vi "진짜 최종.vi"() -> ()   [LabVIEW 2016]
uses:
  <vilib>/DAQmx/write.llb/DAQmx Write (Digital 1D U32 1Chan NSamp).vi
  <vilib>/DAQmx/read.llb/DAQmx Read (Analog 1D Wfm NChan NSamp).vi
  <vilib>/DAQmx/create/channels.llb/DAQmx Create Channel (DO-Digital Output).vi
  <vilib>/DAQmx/configure/timing.llb/DAQmx Timing (Sample Clock).vi
  <vilib>/DAQmx/create/channels.llb/DAQmx Create Channel (AI-Acceleration-Accelerometer).vi
  <vilib>/DAQmx/miscellaneous.llb/DAQmx Fill In Error Info.vi
panel:
  out "Elapsed Time (s) 9":dbl caption="대기상태 경과시간"
  out "1세트점수":i32
  out "0세트점수":i32
  out "몇번째 경기":i32
  out "1터치횟수":i32
  out "0터치횟수":i32
  out "player 1":bool
  out "player 2":bool
  out "0현점수":i32
  out "1현점수":i32
  out "0번 터치":bool
  out "1번 터치":bool
  out "Elapsed Time (s) 8":dbl caption="0 터치인식대기"
  out "Elapsed Time (s) 7":dbl caption="1 터치인식대기"
  out "Elapsed Time (s) 6":dbl caption="1리시브"
  out "Elapsed Time (s)":dbl caption="0리시브"
  out "Elapsed Time (s) 5":dbl caption="0세트승리"
  out "Elapsed Time (s) 4":dbl caption="0번 승리 경과"
  out "Elapsed Time (s) 3":dbl caption="1세트승리"
  out "Elapsed Time (s) 2":dbl caption="1번 승리 경과"
  in  "RESET":bool
  # "HA"
  # "JIWON"
  # "2초 reset"
  # "2초 reset"
  # "2초 reset"
  # "0.05초 reset"
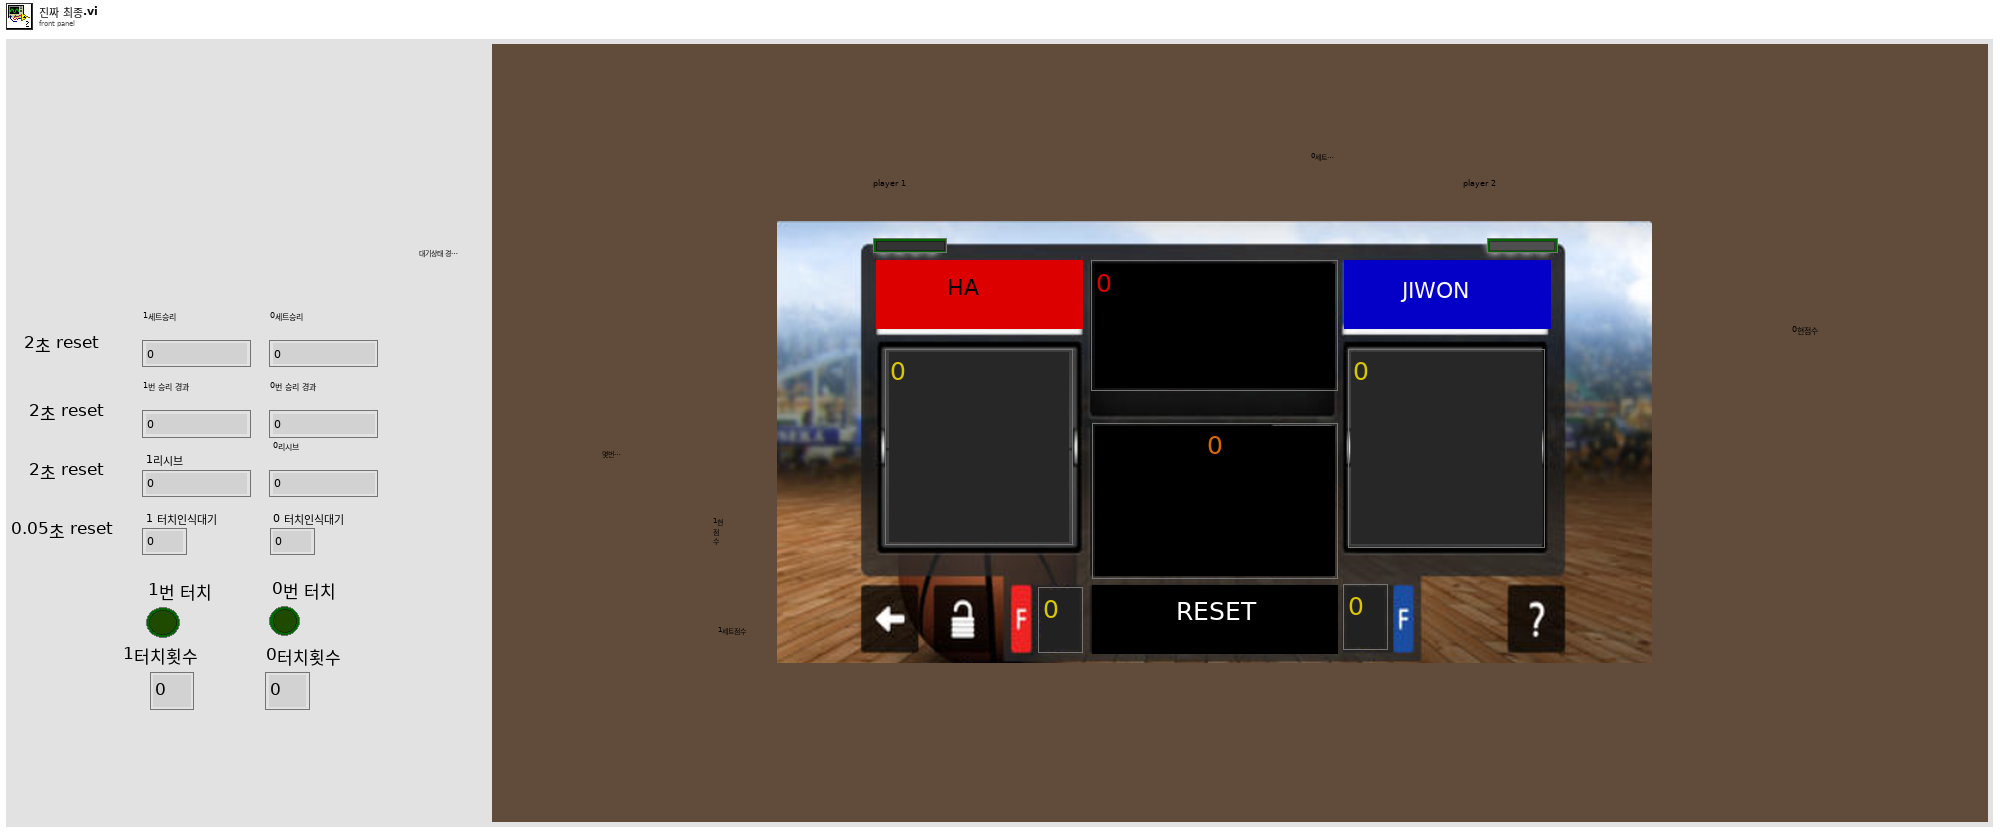
[diagram p1: front panel]
types:
  T1 = typedef "컨트롤 2.ctl" = enum16{"경기끝!", "1세트승리", "0세트승리", "0리시브", "1리시브", "대기", "1번터치", "0번터치", "서브교체", "1번승리", "0번승리"}
  T2 = cluster{"점수":i32[], "몇번째 경기":i32, "LED0":bool, "LED1":bool, "1번터치 횟수":i32, "0현점수":i32, "1현점수":i32, "0번터치 횟수":i32, "0세트점수":i32, "1세트점수":i32, "경과시간":i32, "0세트 이진수점수":u32[], "1세트 이진수점수 ":u32[], "LED1차례":u32[], "LED0차례":u32[]}
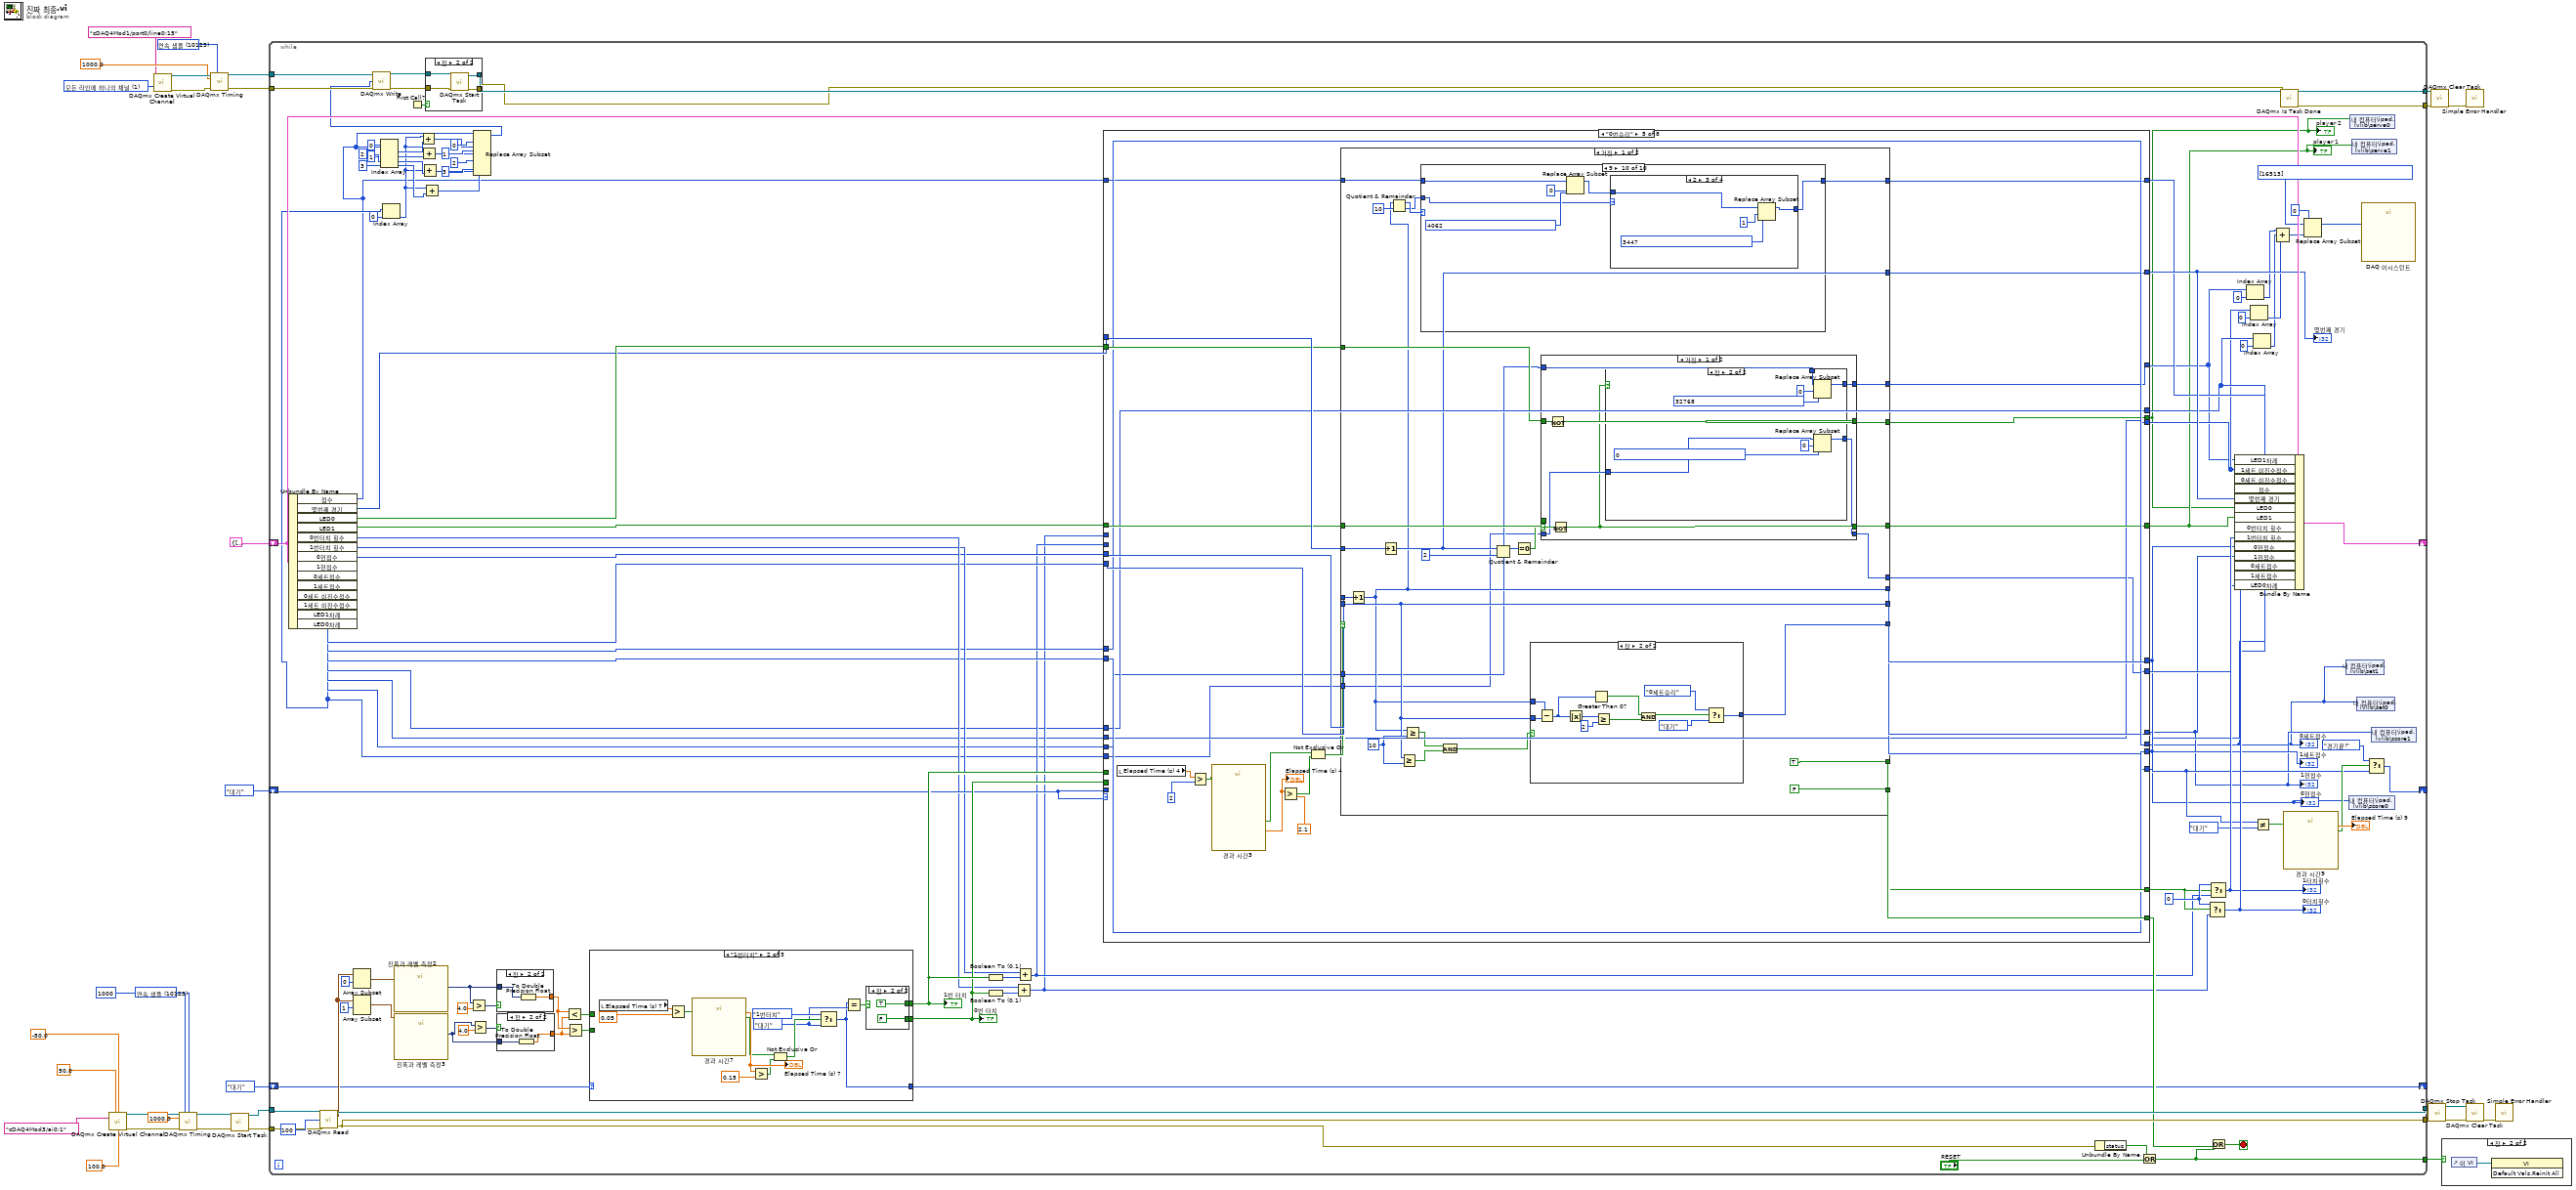
[diagram p0: block diagram]
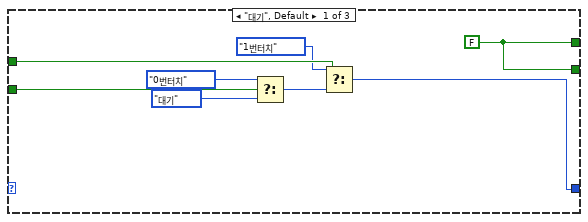
[diagram p2: hidden frame]
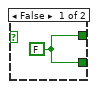
[diagram p3: hidden frame]
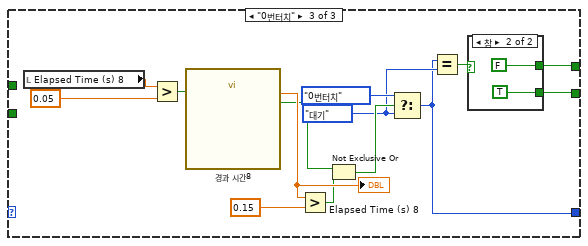
[diagram p4: hidden frame]
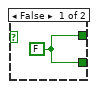
[diagram p5: hidden frame]
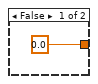
[diagram p6: hidden frame]
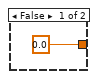
[diagram p7: hidden frame]
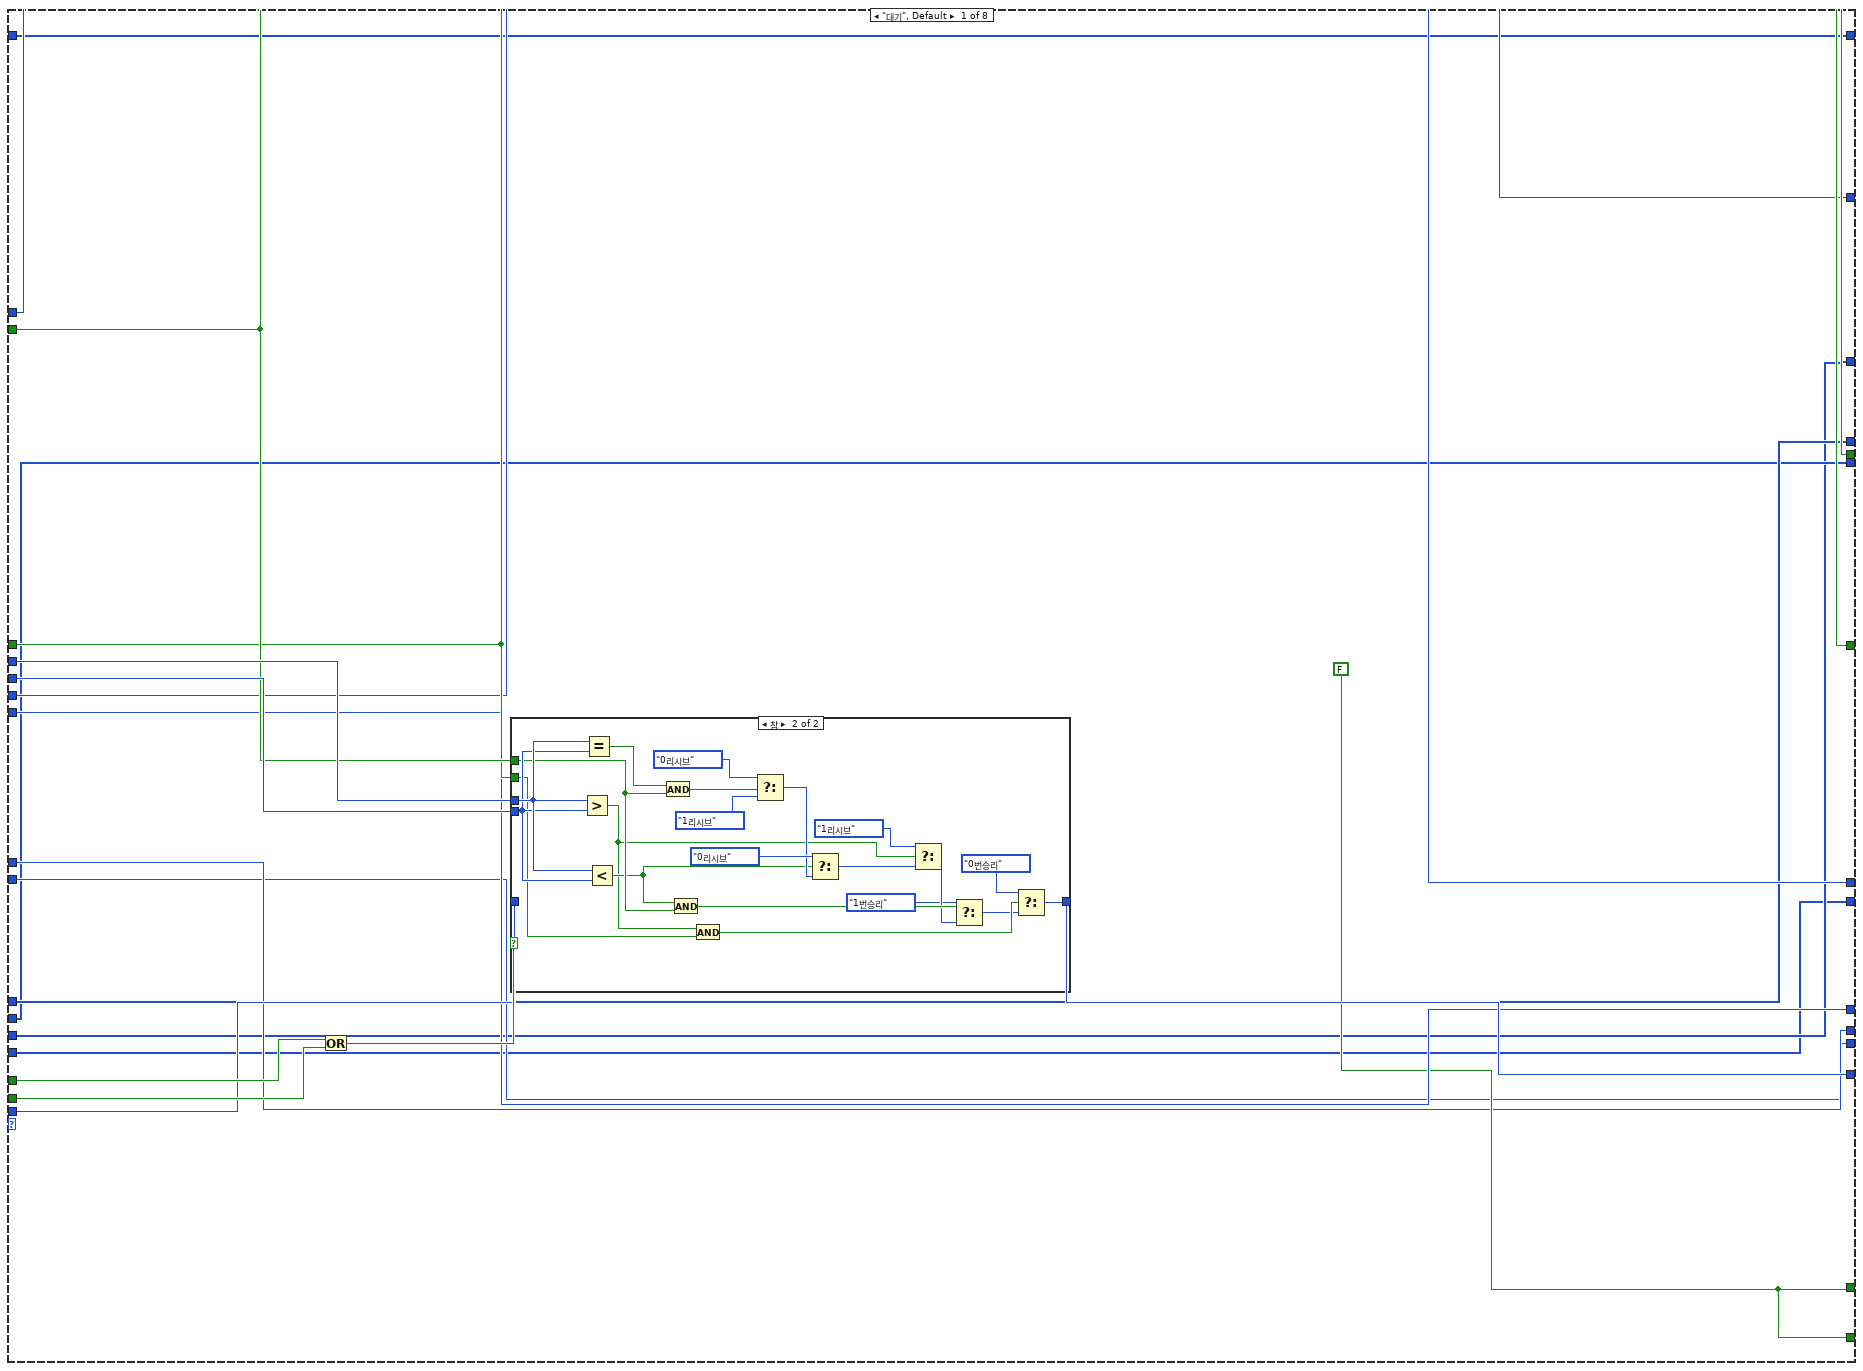
[diagram p8: hidden frame]
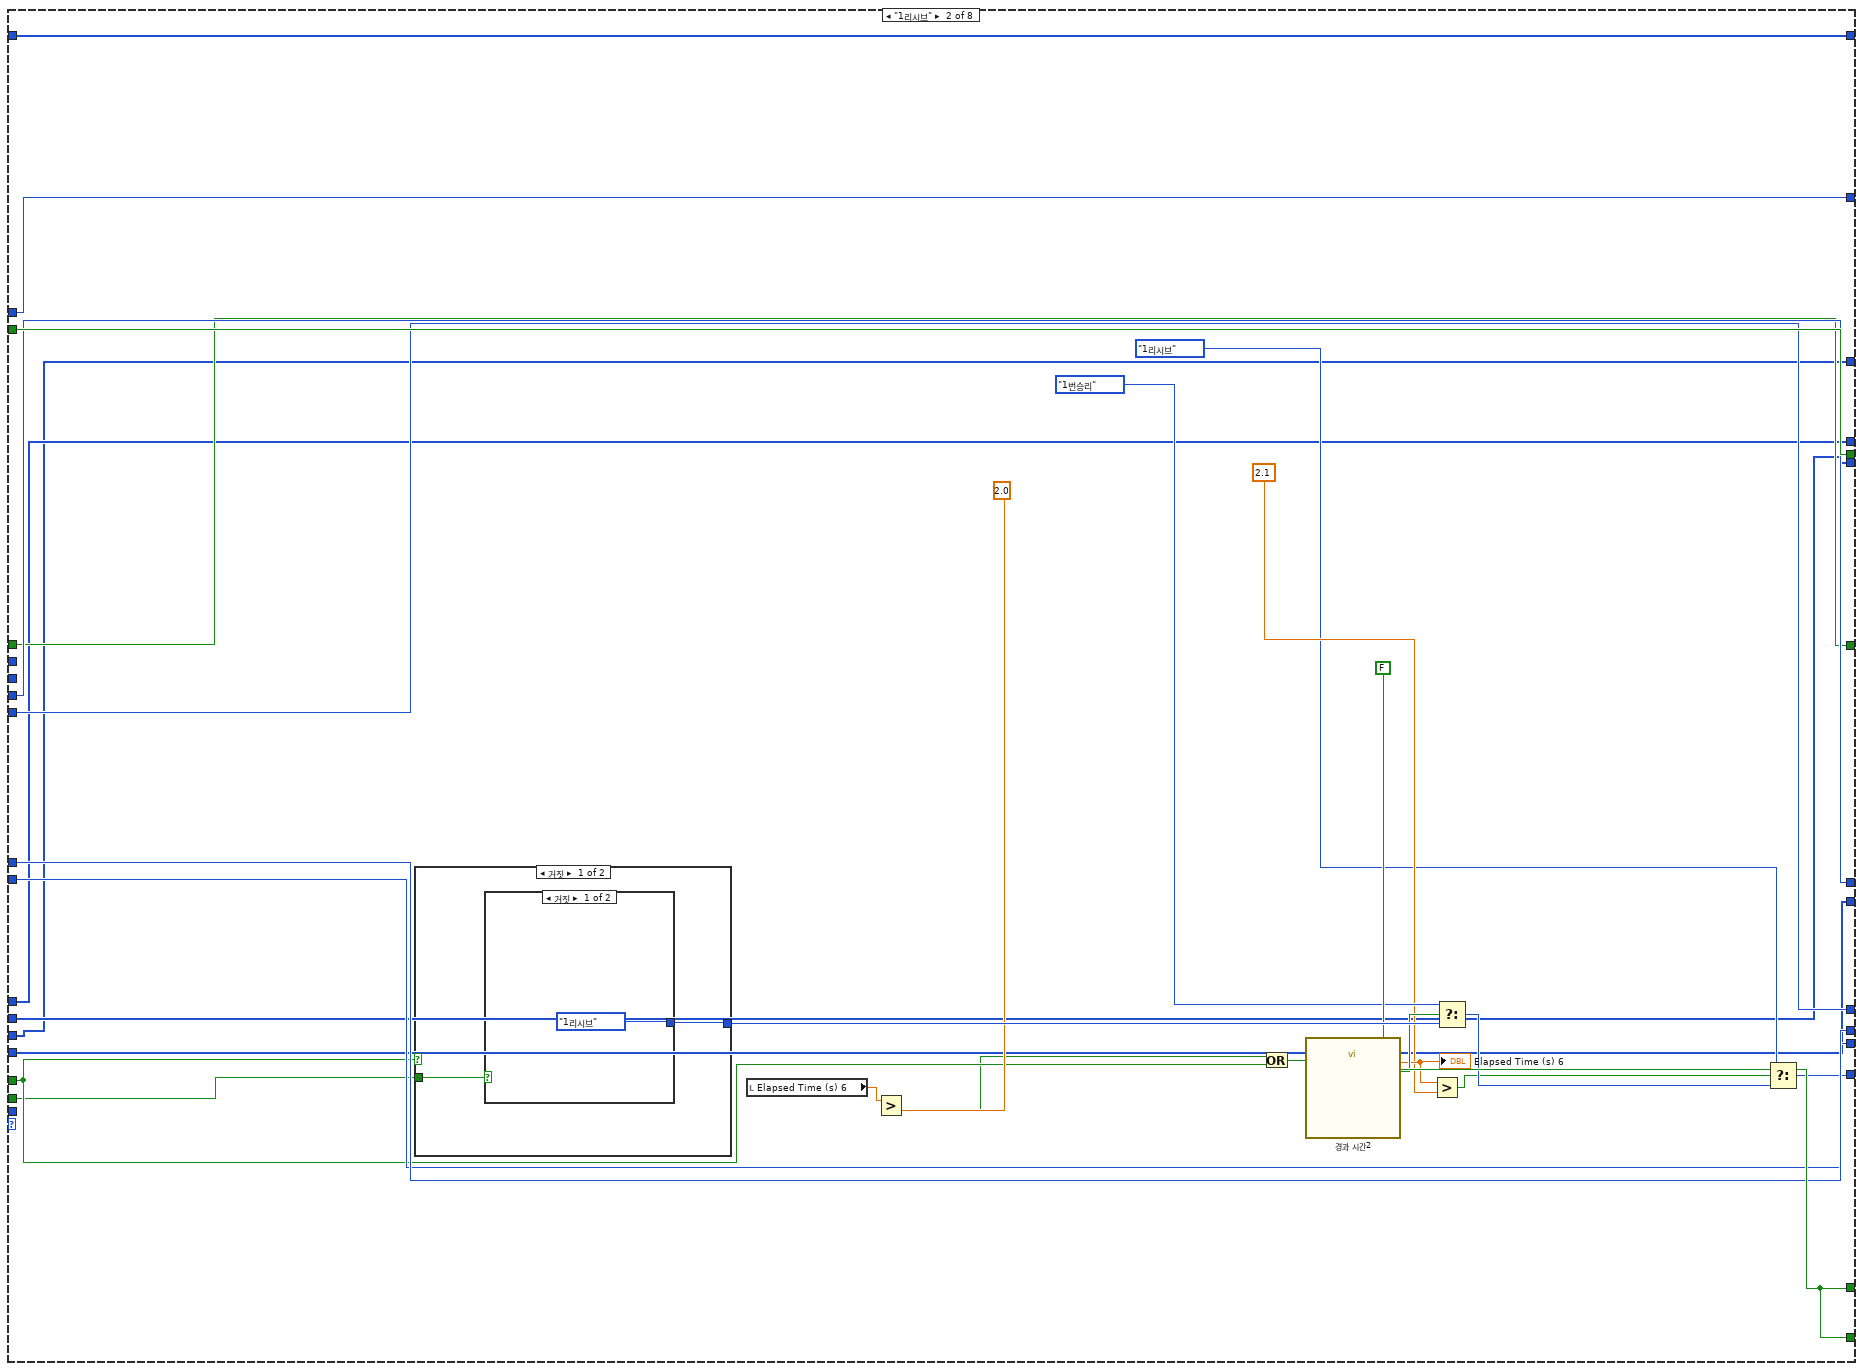
[diagram p10: hidden frame]
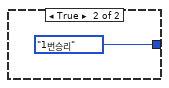
[diagram p11: hidden frame]
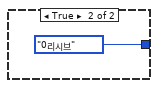
[diagram p12: hidden frame]
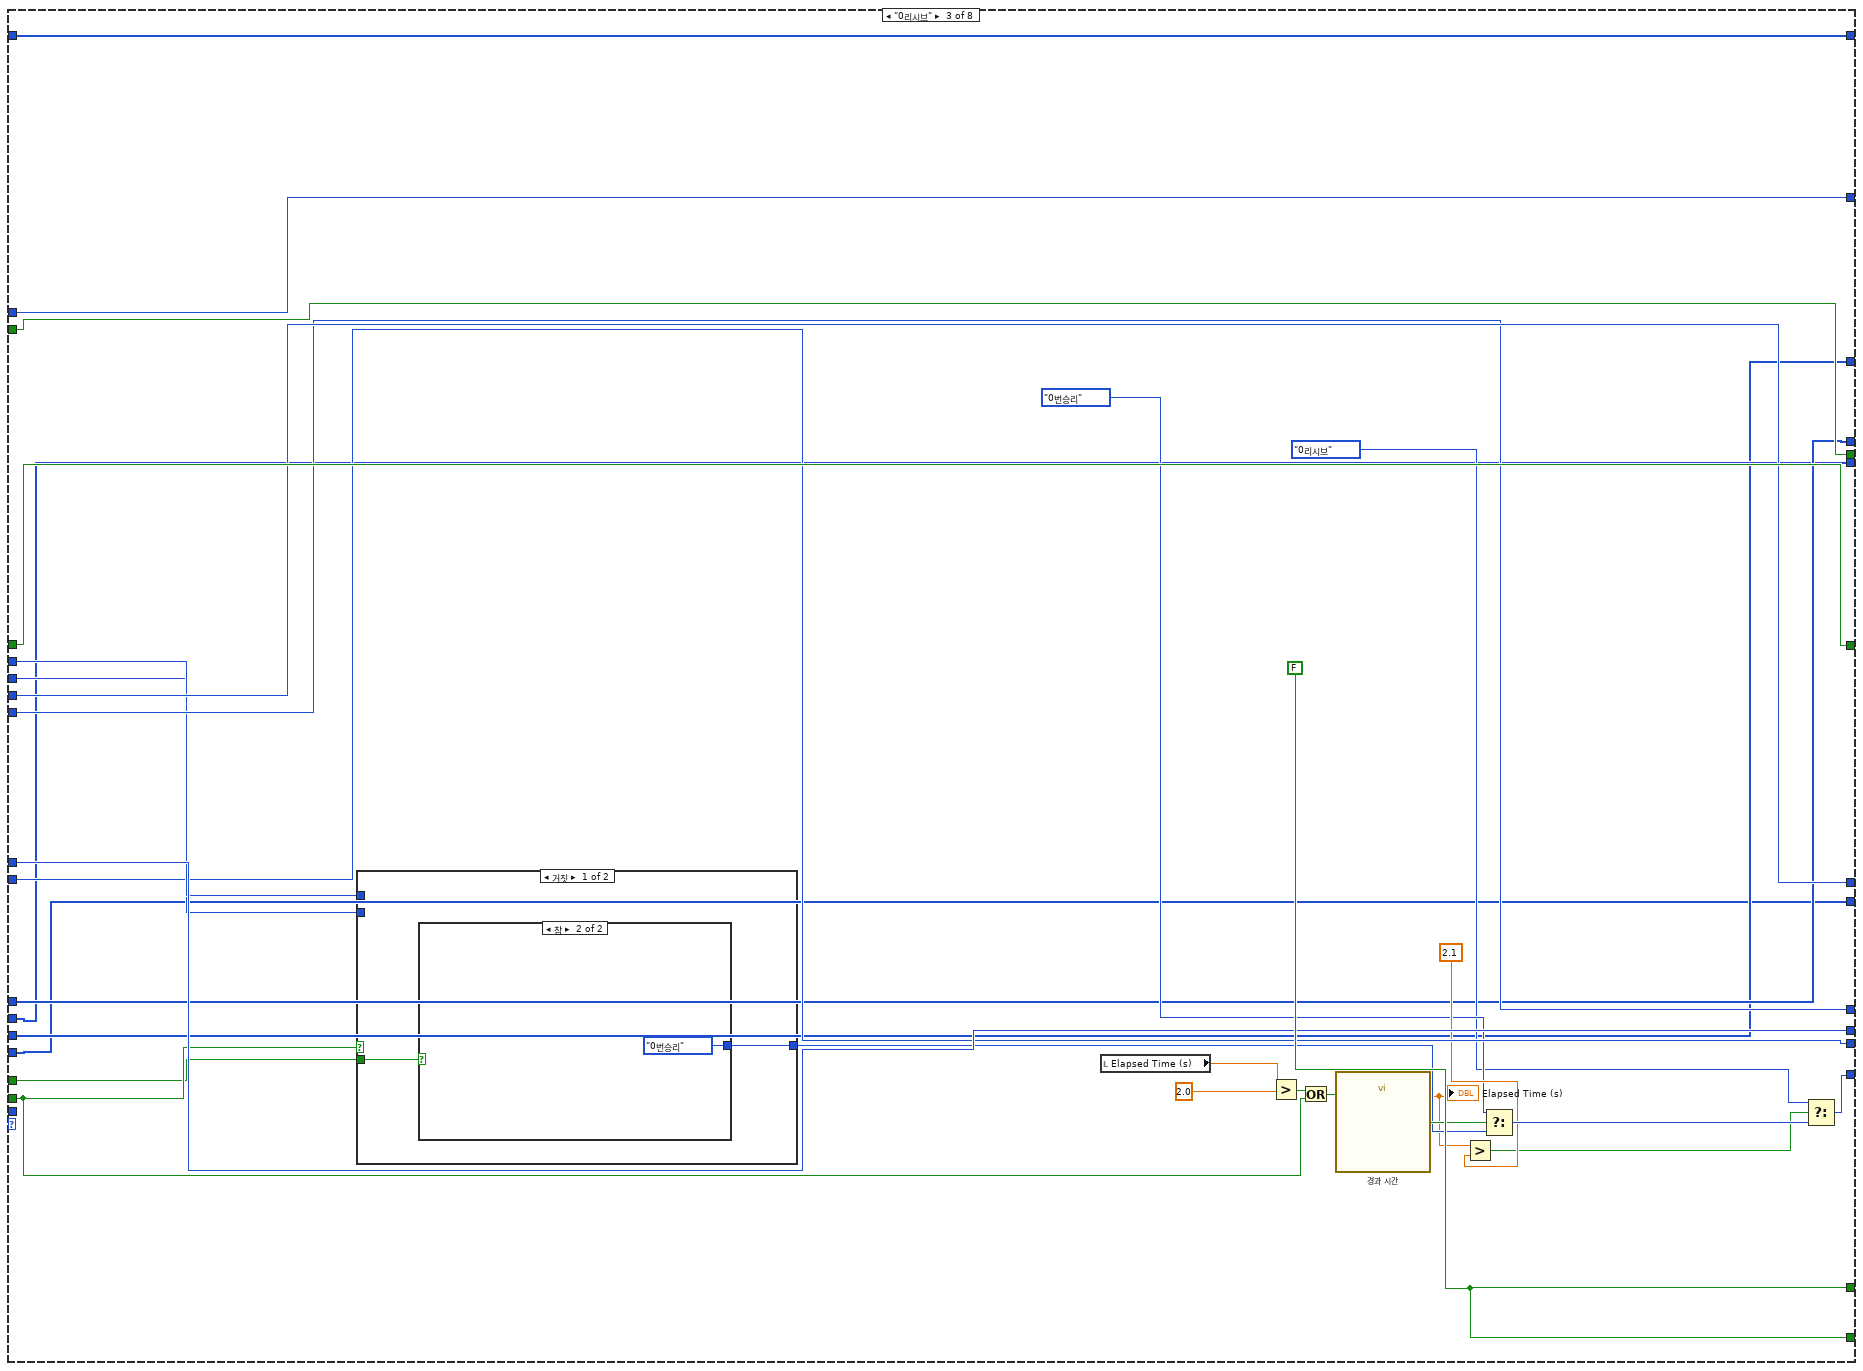
[diagram p13: hidden frame]
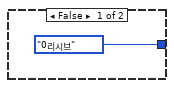
[diagram p14: hidden frame]
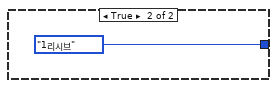
[diagram p15: hidden frame]
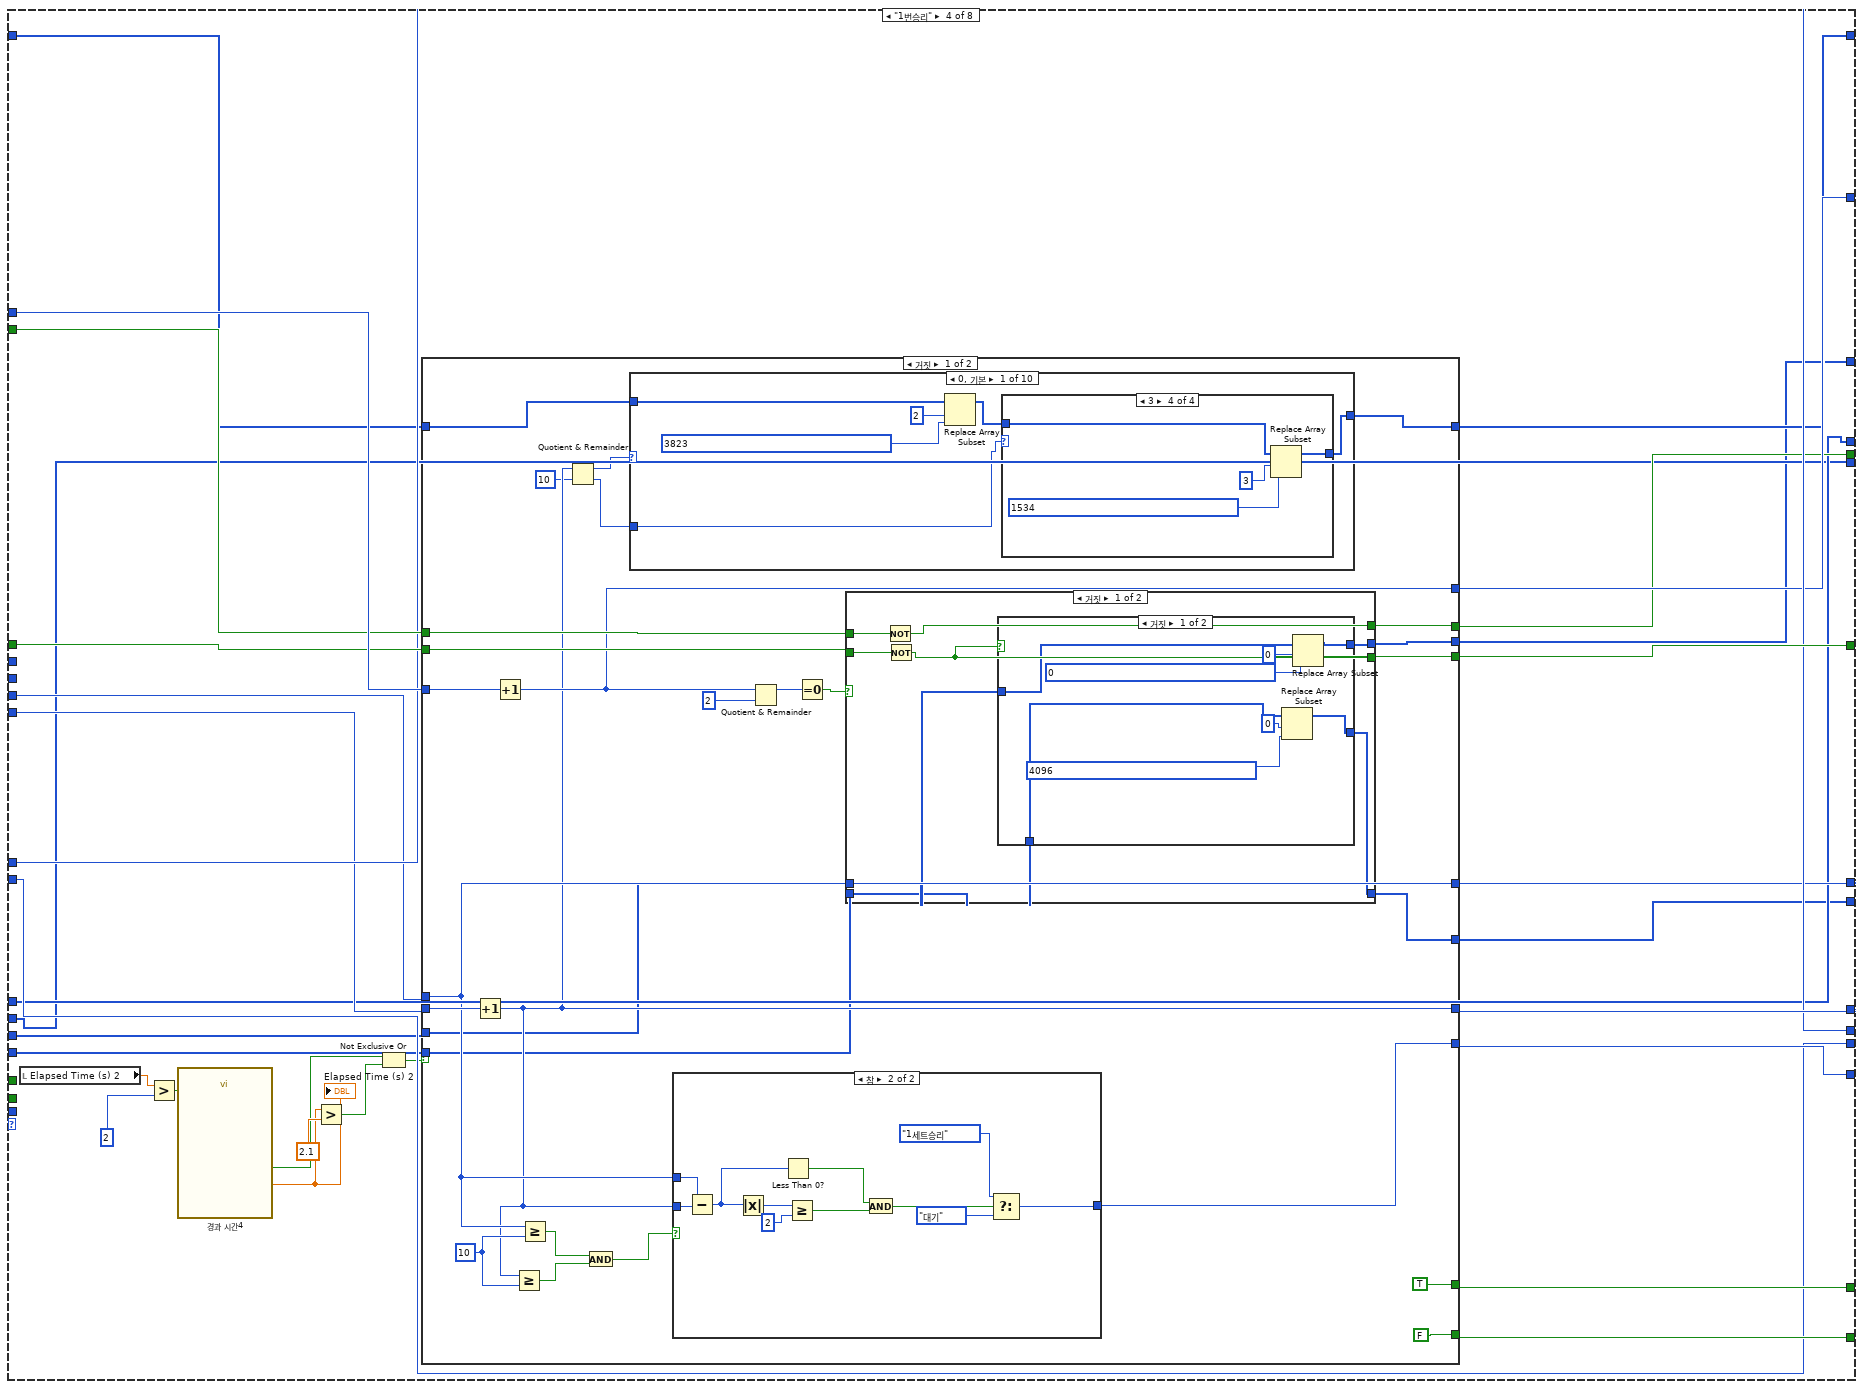
[diagram p16: hidden frame]
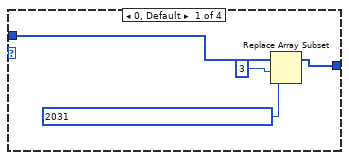
[diagram p17: hidden frame]
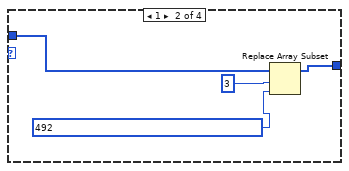
[diagram p18: hidden frame]
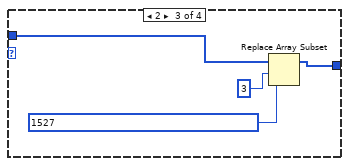
[diagram p19: hidden frame]
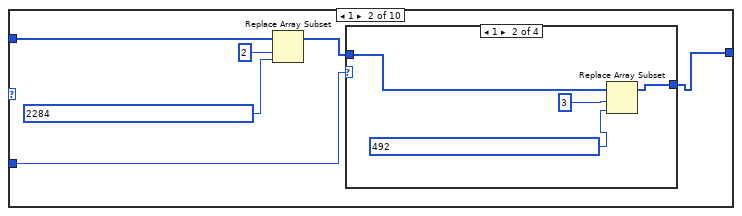
[diagram p20: hidden frame]
diagram:
  w12 = 10123 items=["유한 샘플"=10178, "연속 샘플"=10123, "하드웨어 타이밍에 의한 단일 포인트"=12522] ("sample mode")
  w15 = 1 items=["각 라인에 하나의 채널", "모든 라인에 하나의 채널"] ("line grouping")
  w28 = 10123 items=["유한 샘플"=10178, "연속 샘플"=10123, "하드웨어 타이밍에 의한 단일 포인트"=12522] ("sample mode")
  n1 = call-poly <vilib>:"DAQmx Create Virtual Channel.vi"("maximum value"=50.0 ("최대 가속"), "minimum value"=-50.0 ("최소 가속"), "physical channels"=tag "cDAQ4Mod3/ai0:1" ("아날로그 입력 채널"), "sensitivity"=100.0) -> ("task out"=w32:refnum<k21>, "error out"=w31:errorcluster)  [unwired: 10 in]
  n2 = call-poly <vilib>:"DAQmx Create Virtual Channel.vi"("lines"=tag "cDAQ4Mod1/port0/line0:15", "line grouping"=w15) -> ("task out"=w13:refnum<k21>, "error out"=w14:errorcluster)  [unwired: 12 in]
  n3 = call-poly <vilib>:"DAQmx Timing.vi"("task/channels in"=w32, "sample mode"=w28, "samples per channel"=1000, "rate"=1000.0 ("샘플 속도"), "error in"=w31) -> ("task out"=w30:refnum<k21>, "error out"=w23:errorcluster)  [unwired: 9 in]
  n4 = call-poly <vilib>:"DAQmx Timing.vi"("task/channels in"=w13, "sample mode"=w12, "rate"=1000.0 ("디지털 클럭 속도"), "error in"=w14) -> ("task out"=w6:refnum<k21>, "error out"=w5:errorcluster)  [unwired: 10 in]
  n5 = call <vilib>:"DAQmx Start Task.vi"("task/channels in"=w30, "error in"=w23) -> ("task out"=w22:refnum<k21>, "error out"=w21:errorcluster)  [unwired: 12 in]
  n6 = while {
    tunnel: w22 -> [w143]
    tunnel: w21 -> [w142]
    tunnel: [w141] -> w18
    tunnel: [w136] -> w16
    tunnel: [w132] -> w8
    tunnel: [w131] -> w7
    tunnel: w6 -> [w129]
    tunnel: w5 -> [w130]
    shift-right: [w118] -> _
    shift-left: T2 {"점수"=[4047, 3951, 3823, 2031], "몇번째 경기"=1, "LED0"=TRUE, "LED1"=FALSE, "1번터치 횟수"=0, "0현점수"=0, "1현점수"=0, "0번터치 횟수"=0, "0세트점수"=0, "1세트점수"=0, "경과시간"=0, "0세트 이진수점수"=[16384], "1세트 이진수점수 "=[129], "LED1차례"=[0], "LED0차례"=[4096]} -> [w108]
    shift-right: [w88] -> _
    shift-left: 컨트롤_2."대기" -> [w113]
    tunnel: [w36] -> w2
    shift-right: [w90] -> _
    shift-left: 컨트롤_2."대기" -> [w93]
    stop <- w96 stop-if-true
    w102 = 0
    n7 = Unbundle By Name(w108) -> ("점수"=w43:i32[], "몇번째 경기"=w63:i32, "LED0"=w110:bool, "LED1"=w109:bool, "0번터치 횟수"=w112:i32, "1번터치 횟수"=w111:i32, "0현점수"=w107:i32, "1현점수"=w106:i32, "0세트점수"=w99:i32, "1세트점수"=w98:i32, "0세트 이진수점수"=w80:u32[], "1세트 이진수점수"=w79:u32[], "LED1차례"=w68:u32[], "LED0차례"=w54:u32[])
    n8 = call-poly <vilib>:"DAQmx Read.vi"("task/channels in"=w143, "number of samples per channel"=100 ("루프당 샘플"), "error in"=w142) -> ("task out"=w141:refnum<k21>, "data"=w104:waveform(dbl)[], "error out"=w136:errorcluster)  [unwired: 10 in]
    n9 = Array Subset(array=w104, index=1 ("인덱스")) -> (w138:waveform(dbl)[])  [unwired: 1 in]
    n10 = Array Subset(array=w104, index=0 ("인덱스")) -> (w122:waveform(dbl)[])  [unwired: 1 in]
    n11 = Index Array(array=w43, index #1=0 ("인덱스"), index #2=1 ("인덱스"), index #3=2 ("인덱스"), index #4=3 ("인덱스")) -> (element #1=w61:i32, element #2=w60:i32, element #3=w56:i32, element #4=w55:i32)
    n12 = Index Array(array=w54, index=0 ("인덱스")) -> (element=w52:u32)
    n13 = call "진폭과 레벨 측정2"("Signals"=w122) -> ("Peak to Peak"=w124:dynamicdata)  [unwired: 13 in, 1 out]
    n14 = call "진폭과 레벨 측정3"("Signals"=w138) -> ("Peak to Peak"=w123:dynamicdata)  [unwired: 13 in, 1 out]
    n15 = First Call?() -> (First Call?: T/F=w125:bool)
    n16 = Add(x=w52, y=w61) -> (x+y=w47:u32)
    n17 = Add(x=w52, y=w60) -> (x+y=w46:u32)
    n18 = Add(x=w52, y=w56) -> (x+y=w45:u32)
    n19 = Add(x=w52, y=w55) -> (x+y=w44:u32)
    n20 = Greater?(x=w124, y=4.0) -> (0:w134:dynamicdata)
    n21 = Greater?(x=w123, y=4.0) -> (0:w137:dynamicdata)
    n22 = Replace Array Subset(array=w43, new element #1=w47, index #1=0 ("인덱스"), new element #2=w46, index #2=1 ("인덱스"), new element #3=w45, index #3=2 ("인덱스"), new element #4=w44, index #4=3 ("인덱스")) -> (w42:i32[])
    n23 = call-poly <vilib>:"DAQmx Write.vi"("task/channels in"=w129, "data"=w42, "error in"=w130) -> ("task out"=w128:refnum<k21>, "error out"=w127:errorcluster)  [unwired: 10 in, 1 out]
    n24 = case shown="참" w125 {
      tunnel: w128 -> [w1093 w1097]
      tunnel: w127 -> [w1092 w1096]
      tunnel: [w1092 w1095] -> w81
      tunnel: [w1093 w1094] -> w126
      frame False {
      }
      frame True {
        n25 = call <vilib>:"DAQmx Start Task.vi"("task/channels in"=w1097, "error in"=w1096) -> ("task out"=w1094:refnum<k21>, "error out"=w1095:errorcluster)  [unwired: 12 in]
      }
    }
    n26 = case shown="참" w134 {
      tunnel: w124 -> [_ w191]
      tunnel: [0.0 w192] -> w121
      frame False {
      }
      frame True {
        n27 = To Double Precision Float(number=w191) -> (double precision float=w192:dbl)
      }
    }
    n28 = case shown="참" w137 {
      tunnel: w123 -> [_ w188]
      tunnel: [0.0 w189] -> w120
      frame False {
      }
      frame True {
        n29 = To Double Precision Float(number=w188) -> (double precision float=w189:dbl)
      }
    }
    n30 = Less?(x=w121, y=w120) -> (x < y?=w91:bool)
    n31 = Greater?(x=w121, y=w120) -> (0:w92:bool)
    n32 = case shown="\"1번터치\"" w93 {
      tunnel: [w152 w166 w171] -> w115
      tunnel: [w152 w165 w170] -> w114
      tunnel: w92 -> [w151 _ _]
      tunnel: w91 -> [w149 _ _]
      tunnel: [w145 w153 w172] -> w90
      frame "대기", Default {
        w152 = FALSE
        n33 = Select(t=컨트롤_2."0번터치", s=w151, f=컨트롤_2."대기") -> (s? t:f=w148:T1)
        n34 = Select(t=컨트롤_2."1번터치", s=w149, f=w148) -> (s? t:f=w145:T1)
      }
      frame "1번터치" {
        w154 = 컨트롤_2."대기"
        n35 = local read "Elapsed Time (s) 7"() -> (w164:dbl)
        n36 = Greater?(x=w164, y=0.05) -> (0:w162:bool)
        n37 = call "경과 시간7"("Reset"=w162) -> ("Elapsed Time (s)"=w161:dbl, "Time has Elapsed"=w159:bool)  [unwired: 11 in, 6 out]
        "Elapsed Time (s) 7" <- w161
        n38 = Greater?(x=w161, y=0.15) -> (0:w158:bool)
        n39 = Not Exclusive Or(1:w158, 2:w159) -> (0:w157:bool)
        n40 = Select(t=컨트롤_2."1번터치", s=w157, f=w154) -> (s? t:f=w153:T1)
        n41 = Equal?(x=w153, y=w154) -> (x = y?=w155:bool)
        n42 = case shown="참" w155 {
          tunnel: [w167 TRUE] -> w166
          tunnel: [w167 FALSE] -> w165
          frame False {
            w167 = FALSE
          }
          frame True {
          }
        }
      }
      frame "0번터치" {
        w173 = 컨트롤_2."대기"
        n43 = local read "Elapsed Time (s) 8"() -> (w183:dbl)
        n44 = Greater?(x=w183, y=0.05) -> (0:w181:bool)
        n45 = call "경과 시간8"("Reset"=w181) -> ("Elapsed Time (s)"=w180:dbl, "Time has Elapsed"=w178:bool)  [unwired: 11 in, 6 out]
        "Elapsed Time (s) 8" <- w180
        n46 = Greater?(x=w180, y=0.15) -> (0:w177:bool)
        n47 = Not Exclusive Or(1:w177, 2:w178) -> (0:w176:bool)
        n48 = Select(t=컨트롤_2."0번터치", s=w176, f=w173) -> (s? t:f=w172:T1)
        n49 = Equal?(x=w172, y=w173) -> (x = y?=w174:bool)
        n50 = case shown="참" w174 {
          tunnel: [w184 FALSE] -> w171
          tunnel: [w184 TRUE] -> w170
          frame False {
            w184 = FALSE
          }
          frame True {
          }
        }
      }
    }
    "1번 터치" <- w115
    "0번 터치" <- w114
    n51 = Boolean To (0,1)(Boolean=w115) -> (0, 1=w116:i16)
    n52 = Boolean To (0,1)(Boolean=w114) -> (0, 1=w117:i16)
    n53 = Add(x=w112, y=w117) -> (x+y=w94:i32)
    n54 = Add(x=w111, y=w116) -> (x+y=w95:i32)
    n55 = case shown="\"0번승리\"" w113 {
      tunnel: w63 -> [w203 w258 w297 w333 w665 w988 w1040 w1085]
      tunnel: w115 -> [w212 w252 w282 _ _ _ _ _]
      tunnel: w114 -> [w211 w248 w286 _ _ _ _ _]
      tunnel: w113 -> [w209 _ _ _ _ _ _ _]
      tunnel: [w208 w240 w273 w327 w651 w991 w1041 컨트롤_2."대기"] -> w85
      tunnel: w94 -> [w207 _ w290 _ _ _ _ _]
      tunnel: w95 -> [w206 _ w289 _ _ _ _ _]
      tunnel: w110 -> [w205 w261 w296 w332 w664 w990 w1039 _]
      tunnel: w109 -> [w204 w254 w295 w331 w663 w989 w1038 _]
      tunnel: [w205 w261 w296 w322 w655 w990 w1039 w1080] -> w37
      tunnel: [w204 w254 w295 w330 w654 w989 w1038 w1079] -> w38
      tunnel: w107 -> [w202 w260 w294 w318 w662 w981 w1035 w1084]
      tunnel: w106 -> [w201 w259 w293 w321 w661 w980 w1034 w1083]
      tunnel: [w202 w260 w294 w317 w660 w986 w1037 w1084] -> w40
      tunnel: [w203 w258 w297 w323 w656 w988 w1040 w1085] -> w105
      tunnel: [w200 w257 w292 w328 w657 w987 w1028 FALSE] -> w101
      tunnel: w99 -> [w199 w256 w291 w325 w659 w994 w1044 w1078]
      tunnel: w98 -> [w198 w255 w288 w324 w653 w993 w1043 w1082]
      tunnel: [w199 w256 w291 w325 w659 w992 w1044 w1078] -> w34
      tunnel: [w198 w255 w288 w324 w653 w993 w1042 w1082] -> w41
      tunnel: [w200 w257 w292 w326 w658 w987 w1028 TRUE] -> w97
      tunnel: [w201 w259 w293 w329 w652 w979 w1036 w1083] -> w39
      tunnel: w43 -> [w197 w239 w272 w310 w644 w971 w1021 w1075]
      tunnel: [w197 w239 w272 w309 w643 w972 w1022 w1075] -> w82
      tunnel: w80 -> [w196 w238 w271 w308 w642 w977 w1025 w1074]
      tunnel: [w196 w238 w271 w308 w642 w976 w1025 w1074] -> w76
      tunnel: w79 -> [w195 w237 w270 w307 w641 w975 w1027 w1073]
      tunnel: [w195 w237 w270 w307 w641 w975 w1026 w1073] -> w73
      tunnel: w68 -> [w194 w236 w269 w306 w640 w974 w1024 w1072]
      tunnel: [w194 w236 w269 w305 w637 w974 w1024 w1072] -> w67
      tunnel: w54 -> [w193 w235 w268 w303 w639 w973 w1023 w1071]
      tunnel: [w193 w235 w268 w304 w638 w973 w1023 w1071] -> w64
      frame "대기", Default {
        w200 = FALSE
        n56 = Or(x=w212, y=w211) -> (x .or. y?=w210:bool)
        n57 = case shown="참" w210 {
          tunnel: w209 -> [w213 _]
          tunnel: [w213 w214] -> w208
          tunnel: w207 -> [_ w234]
          tunnel: w206 -> [_ w233]
          tunnel: w205 -> [_ w224]
          tunnel: w204 -> [_ w216]
          frame False {
          }
          frame True {
            n58 = Greater?(x=w234, y=w233) -> (0:w215:bool)
            n59 = Equal?(x=w234, y=w233) -> (x = y?=w232:bool)
            n60 = Less?(x=w234, y=w233) -> (x < y?=w223:bool)
            n61 = And(x=w232, y=w224) -> (x .and. y?=w231:bool)
            n62 = And(x=w223, y=w224) -> (x .and. y?=w222:bool)
            n63 = And(x=w215, y=w216) -> (x .and. y?=w218:bool)
            n64 = Select(t=컨트롤_2."0리시브", s=w231, f=컨트롤_2."1리시브") -> (s? t:f=w226:T1)
            n65 = Select(t=컨트롤_2."0리시브", s=w223, f=w226) -> (s? t:f=w227:T1)
            n66 = Select(t=컨트롤_2."1리시브", s=w215, f=w227) -> (s? t:f=w221:T1)
            n67 = Select(t=컨트롤_2."1번승리", s=w222, f=w221) -> (s? t:f=w217:T1)
            n68 = Select(t=컨트롤_2."0번승리", s=w218, f=w217) -> (s? t:f=w214:T1)
          }
        }
      }
      frame "1리시브" {
        w257 = FALSE
        n69 = case shown="거짓" w252 {
          tunnel: [w264 컨트롤_2."0리시브"] -> w262
          tunnel: w248 -> [w263 _]
          frame False {
            n70 = case shown="거짓" w263 {
              tunnel: [컨트롤_2."1리시브" 컨트롤_2."1번승리"] -> w264
              frame False {
              }
              frame True {
              }
            }
          }
          frame True {
          }
        }
        n71 = local read "Elapsed Time (s) 6"() -> (w249:dbl)
        n72 = Greater?(x=w249, y=2.0) -> (0:w251:bool)
        n73 = Or(x=w251, y=w252) -> (x .or. y?=w250:bool)
        n74 = call "경과 시간2"("Reset"=w250) -> ("Elapsed Time (s)"=w244:dbl, "Time has Elapsed"=w246:bool)  [unwired: 11 in, 6 out]
        "Elapsed Time (s) 6" <- w244
        n75 = Greater?(x=w244, y=2.1) -> (0:w242:bool)
        n76 = Select(t=컨트롤_2."1번승리", s=w246, f=w262) -> (s? t:f=w245:T1)
        n77 = Select(t=컨트롤_2."1리시브", s=w242, f=w245) -> (s? t:f=w240:T1)
      }
      frame "0리시브" {
        w292 = FALSE
        n78 = case shown="거짓" w286 {
          tunnel: [w299 컨트롤_2."1리시브"] -> w276
          tunnel: w290 -> [_ _]
          tunnel: w289 -> [_ _]
          tunnel: w282 -> [w298 _]
          frame False {
            n79 = case shown="참" w298 {
              tunnel: [컨트롤_2."0리시브" 컨트롤_2."0번승리"] -> w299
              frame False {
              }
              frame True {
              }
            }
          }
          frame True {
          }
        }
        n80 = local read "Elapsed Time (s)"() -> (w283:dbl)
        n81 = Greater?(x=w283, y=2.0) -> (0:w285:bool)
        n82 = Or(x=w285, y=w286) -> (x .or. y?=w284:bool)
        n83 = call "경과 시간"("Reset"=w284) -> ("Elapsed Time (s)"=w275:dbl, "Time has Elapsed"=w278:bool)  [unwired: 11 in, 6 out]
        "Elapsed Time (s)" <- w275
        n84 = Greater?(x=w275, y=2.1) -> (0:w279:bool)
        n85 = Select(t=컨트롤_2."0번승리", s=w278, f=w276) -> (s? t:f=w281:T1)
        n86 = Select(t=컨트롤_2."0리시브", s=w279, f=w281) -> (s? t:f=w273:T1)
      }
      frame "1번승리" {
        n87 = local read "Elapsed Time (s) 2"() -> (w316:dbl)
        n88 = Greater?(x=w316, y=2) -> (0:w319:bool)
        n89 = call "경과 시간4"("Reset"=w319) -> ("Elapsed Time (s)"=w314:dbl, "Time has Elapsed"=w312:bool)  [unwired: 11 in, 6 out]
        "Elapsed Time (s) 2" <- w314
        n90 = Greater?(x=w314, y=2.1) -> (0:w313:bool)
        n91 = Not Exclusive Or(1:w313, 2:w312) -> (0:w311:bool)
        n92 = case shown="거짓" w311 {
          tunnel: w333 -> [w361 w633]
          tunnel: w332 -> [w360 w632]
          tunnel: w331 -> [w359 w631]
          tunnel: [w358 w631] -> w330
          tunnel: [w341 w634] -> w329
          tunnel: [TRUE w635] -> w328
          tunnel: [w345 컨트롤_2."1번승리"] -> w327
          tunnel: [FALSE w635] -> w326
          tunnel: [w355 w633] -> w323
          tunnel: [w351 w632] -> w322
          tunnel: w321 -> [w347 w634]
          tunnel: w318 -> [w346 w630]
          tunnel: [w346 w630] -> w317
          tunnel: w310 -> [w343 w629]
          tunnel: [w342 w629] -> w309
          tunnel: w306 -> [w337 w628]
          tunnel: [w336 w628] -> w305
          tunnel: [w335 w627] -> w304
          tunnel: w303 -> [w334 w627]
          frame False {
            w350 = 10
            n93 = Increment(x=w347) -> (x+1=w341:i32)
            n94 = Increment(x=w361) -> (x+1=w355:i32)
            n95 = Greater Or Equal?(x=w341, y=w350) -> (x >= y?=w348:bool)
            n96 = Greater Or Equal?(x=w346, y=w350) -> (x >= y?=w349:bool)
            n97 = Quotient & Remainder(x=w341, y=10) -> (x-y*floor(x/y)=w339:i32, floor(x/y)=w338:i32)
            n98 = And(x=w349, y=w348) -> (x .and. y?=w344:bool)
            n99 = case shown="0, 기본" w339 {
              tunnel: w343 -> [w366 w388 w409 w431 w453 w475 w497 w519 w541 w563]
              tunnel: [w362 w384 w406 w430 w452 w474 w494 w518 w540 w562] -> w342
              tunnel: w338 -> [w363 w385 w407 w428 w450 w472 w495 w516 w538 w560]
              frame 0, Default {
                n100 = Replace Array Subset(array=w366, new element=3823 ("현점수"), index=2 ("인덱스")) -> (w364:i32[])
                n101 = case shown="3" w363 {
                  tunnel: w364 -> [w370 w374 w378 w382]
                  tunnel: [w369 w373 w377 w381] -> w362
                  frame 0, Default {
                    n102 = Replace Array Subset(array=w370, new element=2031 ("현점수"), index=3 ("인덱스")) -> (w369:i32[])
                  }
                  frame 1 {
                    n103 = Replace Array Subset(array=w374, new element=492 ("현점수"), index=3 ("인덱스")) -> (w373:i32[])
                  }
                  frame 2 {
                    n104 = Replace Array Subset(array=w378, new element=1527 ("현점수"), index=3 ("인덱스")) -> (w377:i32[])
                  }
                  frame 3 {
                    n105 = Replace Array Subset(array=w382, new element=1534 ("현점수"), index=3 ("인덱스")) -> (w381:i32[])
                  }
                }
              }
              frame 1 {
                n106 = Replace Array Subset(array=w388, new element=2284 ("현점수"), index=2 ("인덱스")) -> (w386:i32[])
                n107 = case shown="1" w385 {
                  tunnel: w386 -> [w392 w396 w400 w404]
                  tunnel: [w391 w395 w399 w403] -> w384
                  frame 0, Default {
                    n108 = Replace Array Subset(array=w392, new element=2031 ("현점수"), index=3 ("인덱스")) -> (w391:i32[])
                  }
                  frame 1 {
                    n109 = Replace Array Subset(array=w396, new element=492 ("현점수"), index=3 ("인덱스")) -> (w395:i32[])
                  }
                  frame 2 {
                    n110 = Replace Array Subset(array=w400, new element=1527 ("현점수"), index=3 ("인덱스")) -> (w399:i32[])
                  }
                  frame 3 {
                    n111 = Replace Array Subset(array=w404, new element=1534 ("현점수"), index=3 ("인덱스")) -> (w403:i32[])
                  }
                }
              }
              frame 2 {
                n112 = Replace Array Subset(array=w409, new element=3319 ("현점수"), index=2 ("인덱스")) -> (w408:i32[])
                n113 = case shown="1" w407 {
                  tunnel: w408 -> [w414 w418 w422 w426]
                  tunnel: [w413 w417 w421 w425] -> w406
                  frame 0, Default {
                    n114 = Replace Array Subset(array=w414, new element=2031 ("현점수"), index=3 ("인덱스")) -> (w413:i32[])
                  }
                  frame 1 {
                    n115 = Replace Array Subset(array=w418, new element=492 ("현점수"), index=3 ("인덱스")) -> (w417:i32[])
                  }
                  frame 2 {
                    n116 = Replace Array Subset(array=w422, new element=1527 ("현점수"), index=3 ("인덱스")) -> (w421:i32[])
                  }
                  frame 3 {
                    n117 = Replace Array Subset(array=w426, new element=1534 ("현점수"), index=3 ("인덱스")) -> (w425:i32[])
                  }
                }
              }
              frame 3 {
                n118 = Replace Array Subset(array=w431, new element=3326 ("현점수"), index=2 ("인덱스")) -> (w429:i32[])
                n119 = case shown="1" w428 {
                  tunnel: w429 -> [w436 w440 w444 w448]
                  tunnel: [w435 w439 w443 w447] -> w430
                  frame 0, Default {
                    n120 = Replace Array Subset(array=w436, new element=2031 ("현점수"), index=3 ("인덱스")) -> (w435:i32[])
                  }
                  frame 1 {
                    n121 = Replace Array Subset(array=w440, new element=492 ("현점수"), index=3 ("인덱스")) -> (w439:i32[])
                  }
                  frame 2 {
                    n122 = Replace Array Subset(array=w444, new element=1527 ("현점수"), index=3 ("인덱스")) -> (w443:i32[])
                  }
                  frame 3 {
                    n123 = Replace Array Subset(array=w448, new element=1534 ("현점수"), index=3 ("인덱스")) -> (w447:i32[])
                  }
                }
              }
              frame 4 {
                n124 = Replace Array Subset(array=w453, new element=2812 ("현점수"), index=2 ("인덱스")) -> (w451:i32[])
                n125 = case shown="1" w450 {
                  tunnel: w451 -> [w458 w462 w466 w470]
                  tunnel: [w457 w461 w465 w469] -> w452
                  frame 0, Default {
                    n126 = Replace Array Subset(array=w458, new element=2031 ("현점수"), index=3 ("인덱스")) -> (w457:i32[])
                  }
                  frame 1 {
                    n127 = Replace Array Subset(array=w462, new element=492 ("현점수"), index=3 ("인덱스")) -> (w461:i32[])
                  }
                  frame 2 {
                    n128 = Replace Array Subset(array=w466, new element=1527 ("현점수"), index=3 ("인덱스")) -> (w465:i32[])
                  }
                  frame 3 {
                    n129 = Replace Array Subset(array=w470, new element=1534 ("현점수"), index=3 ("인덱스")) -> (w469:i32[])
                  }
                }
              }
              frame 5 {
                n130 = Replace Array Subset(array=w475, new element=3774 ("현점수"), index=2 ("인덱스")) -> (w473:i32[])
                n131 = case shown="1" w472 {
                  tunnel: w473 -> [w480 w484 w488 w492]
                  tunnel: [w479 w483 w487 w491] -> w474
                  frame 0, Default {
                    n132 = Replace Array Subset(array=w480, new element=2031 ("현점수"), index=3 ("인덱스")) -> (w479:i32[])
                  }
                  frame 1 {
                    n133 = Replace Array Subset(array=w484, new element=492 ("현점수"), index=3 ("인덱스")) -> (w483:i32[])
                  }
                  frame 2 {
                    n134 = Replace Array Subset(array=w488, new element=1527 ("현점수"), index=3 ("인덱스")) -> (w487:i32[])
                  }
                  frame 3 {
                    n135 = Replace Array Subset(array=w492, new element=1534 ("현점수"), index=3 ("인덱스")) -> (w491:i32[])
                  }
                }
              }
              frame 6 {
                n136 = Replace Array Subset(array=w497, new element=3775 ("현점수"), index=2 ("인덱스")) -> (w496:i32[])
                n137 = case shown="1" w495 {
                  tunnel: w496 -> [w502 w506 w510 w514]
                  tunnel: [w501 w505 w509 w513] -> w494
                  frame 0, Default {
                    n138 = Replace Array Subset(array=w502, new element=2031 ("현점수"), index=3 ("인덱스")) -> (w501:i32[])
                  }
                  frame 1 {
                    n139 = Replace Array Subset(array=w506, new element=492 ("현점수"), index=3 ("인덱스")) -> (w505:i32[])
                  }
                  frame 2 {
                    n140 = Replace Array Subset(array=w510, new element=1527 ("현점수"), index=3 ("인덱스")) -> (w509:i32[])
                  }
                  frame 3 {
                    n141 = Replace Array Subset(array=w514, new element=1534 ("현점수"), index=3 ("인덱스")) -> (w513:i32[])
                  }
                }
              }
              frame 7 {
                n142 = Replace Array Subset(array=w519, new element=3820 ("현점수"), index=2 ("인덱스")) -> (w517:i32[])
                n143 = case shown="1" w516 {
                  tunnel: w517 -> [w524 w528 w532 w536]
                  tunnel: [w523 w527 w531 w535] -> w518
                  frame 0, Default {
                    n144 = Replace Array Subset(array=w524, new element=2031 ("현점수"), index=3 ("인덱스")) -> (w523:i32[])
                  }
                  frame 1 {
                    n145 = Replace Array Subset(array=w528, new element=492 ("현점수"), index=3 ("인덱스")) -> (w527:i32[])
                  }
                  frame 2 {
                    n146 = Replace Array Subset(array=w532, new element=1527 ("현점수"), index=3 ("인덱스")) -> (w531:i32[])
                  }
                  frame 3 {
                    n147 = Replace Array Subset(array=w536, new element=1534 ("현점수"), index=3 ("인덱스")) -> (w535:i32[])
                  }
                }
              }
              frame 8 {
                n148 = Replace Array Subset(array=w541, new element=3839 ("현점수"), index=2 ("인덱스")) -> (w539:i32[])
                n149 = case shown="1" w538 {
                  tunnel: w539 -> [w546 w550 w554 w558]
                  tunnel: [w545 w549 w553 w557] -> w540
                  frame 0, Default {
                    n150 = Replace Array Subset(array=w546, new element=2031 ("현점수"), index=3 ("인덱스")) -> (w545:i32[])
                  }
                  frame 1 {
                    n151 = Replace Array Subset(array=w550, new element=492 ("현점수"), index=3 ("인덱스")) -> (w549:i32[])
                  }
                  frame 2 {
                    n152 = Replace Array Subset(array=w554, new element=1527 ("현점수"), index=3 ("인덱스")) -> (w553:i32[])
                  }
                  frame 3 {
                    n153 = Replace Array Subset(array=w558, new element=1534 ("현점수"), index=3 ("인덱스")) -> (w557:i32[])
                  }
                }
              }
              frame 9 {
                n154 = Replace Array Subset(array=w563, new element=3838 ("현점수"), index=2 ("인덱스")) -> (w561:i32[])
                n155 = case shown="1" w560 {
                  tunnel: w561 -> [w568 w572 w576 w580]
                  tunnel: [w567 w571 w575 w579] -> w562
                  frame 0, Default {
                    n156 = Replace Array Subset(array=w568, new element=2031 ("현점수"), index=3 ("인덱스")) -> (w567:i32[])
                  }
                  frame 1 {
                    n157 = Replace Array Subset(array=w572, new element=492 ("현점수"), index=3 ("인덱스")) -> (w571:i32[])
                  }
                  frame 2 {
                    n158 = Replace Array Subset(array=w576, new element=1527 ("현점수"), index=3 ("인덱스")) -> (w575:i32[])
                  }
                  frame 3 {
                    n159 = Replace Array Subset(array=w580, new element=1534 ("현점수"), index=3 ("인덱스")) -> (w579:i32[])
                  }
                }
              }
            }
            n160 = case shown="참" w344 {
              tunnel: w341 -> [w583 w590]
              tunnel: w346 -> [_ w591]
              tunnel: [w582 w592] -> w345
              frame False {
                n161 = Equal?(x=w583, y=11) -> (x = y?=w584:bool)
                n162 = case shown="거짓" w584 {
                  tunnel: [컨트롤_2."대기" 컨트롤_2."1세트승리"] -> w582
                  frame False {
                  }
                  frame True {
                  }
                }
              }
              frame True {
                n163 = Subtract(x=w591, y=w590) -> (x-y=w594:i32)
                n164 = Absolute Value(x=w594) -> (abs(x)=w593:i32)
                n165 = Less Than 0?(x=w594) -> (x < 0?=w597:bool)
                n166 = Greater Or Equal?(x=w593, y=2) -> (x >= y?=w589:bool)
                n167 = And(x=w597, y=w589) -> (x .and. y?=w596:bool)
                n168 = Select(t=컨트롤_2."1세트승리", s=w596, f=컨트롤_2."대기") -> (s? t:f=w592:T1)
              }
            }
            n169 = Quotient & Remainder(x=w355, y=2) -> (x-y*floor(x/y)=w353:i32)  [unwired: 1 out]
            n170 = Equal To 0?(x=w353) -> (x = 0?=w352:bool)
            n171 = case shown="거짓" w352 {
              tunnel: w360 -> [w606 w626]
              tunnel: w359 -> [w605 w625]
              tunnel: [w602 w626] -> w351
              tunnel: [w601 w625] -> w358
              tunnel: w337 -> [w603 w624]
              tunnel: [w604 w624] -> w336
              tunnel: [w599 w623] -> w335
              tunnel: w334 -> [w600 w623]
              frame False {
                n172 = Not(x=w606) -> (.not. x?=w602:bool)
                n173 = Not(x=w605) -> (.not. x?=w601:bool)
                n174 = case shown="거짓" w601 {
                  tunnel: w603 -> [w612 w620]
                  tunnel: [w611 w619] -> w604
                  tunnel: w600 -> [w608 w616]
                  tunnel: [w607 w615] -> w599
                  frame False {
                    n175 = Replace Array Subset(array=w608, new element=u32 4096 ("Waveform"), index=0 ("인덱스")) -> (w607:u32[])
                    n176 = Replace Array Subset(array=w612, new element=u32 0 ("새 원소/부분배열"), index=0 ("인덱스")) -> (w611:u32[])
                  }
                  frame True {
                    n177 = Replace Array Subset(array=w620, new element=u32 32768 ("새 원소/부분배열"), index=0 ("인덱스")) -> (w619:u32[])
                    n178 = Replace Array Subset(array=w616, new element=u32 0 ("Waveform"), index=0 ("인덱스")) -> (w615:u32[])
                  }
                }
              }
              frame True {
              }
            }
          }
          frame True {
            w635 = FALSE
          }
        }
      }
      frame "0번승리" {
        n179 = local read "Elapsed Time (s) 4"() -> (w650:dbl)
        n180 = Greater?(x=w650, y=2) -> (0:w667:bool)
        n181 = call "경과 시간3"("Reset"=w667) -> ("Elapsed Time (s)"=w646:dbl, "Time has Elapsed"=w647:bool)  [unwired: 11 in, 6 out]
        "Elapsed Time (s) 4" <- w646
        n182 = Greater?(x=w646, y=2.1) -> (0:w648:bool)
        n183 = Not Exclusive Or(1:w648, 2:w647) -> (0:w645:bool)
        n184 = case shown="거짓" w645 {
          tunnel: w665 -> [w695 w967]
          tunnel: w664 -> [w694 w966]
          tunnel: w663 -> [w693 w965]
          tunnel: [w692 w965] -> w654
          tunnel: [w678 w968] -> w652
          tunnel: [TRUE w969] -> w657
          tunnel: [w680 컨트롤_2."0번승리"] -> w651
          tunnel: [FALSE w969] -> w658
          tunnel: [w689 w967] -> w656
          tunnel: [w685 w966] -> w655
          tunnel: w661 -> [w678 w968]
          tunnel: w662 -> [w681 w964]
          tunnel: [w674 w964] -> w660
          tunnel: w644 -> [w677 w963]
          tunnel: [w676 w963] -> w643
          tunnel: [w671 w961] -> w638
          tunnel: [w668 w962] -> w637
          tunnel: w640 -> [w670 w962]
          tunnel: w639 -> [w669 w961]
          frame False {
            w684 = 10
            n185 = Increment(x=w681) -> (x+1=w674:i32)
            n186 = Increment(x=w695) -> (x+1=w689:i32)
            n187 = Quotient & Remainder(x=w674, y=10) -> (x-y*floor(x/y)=w673:i32, floor(x/y)=w672:i32)
            n188 = Greater Or Equal?(x=w678, y=w684) -> (x >= y?=w682:bool)
            n189 = Greater Or Equal?(x=w674, y=w684) -> (x >= y?=w683:bool)
            n190 = case shown="9" w673 {
              tunnel: w677 -> [w700 w722 w743 w765 w787 w809 w831 w853 w875 w897]
              tunnel: [w697 w718 w741 w763 w785 w807 w829 w851 w873 w895] -> w676
              tunnel: w672 -> [w696 w720 w740 w762 w784 w806 w828 w850 w872 w894]
              frame 0, Default {
                n191 = Replace Array Subset(array=w700, new element=4047 ("현점수"), index=0 ("인덱스")) -> (w698:i32[])
                n192 = case shown="3" w696 {
                  tunnel: w698 -> [w704 w708 w712 w716]
                  tunnel: [w703 w707 w711 w715] -> w697
                  frame 0, Default {
                    n193 = Replace Array Subset(array=w704, new element=3951 ("현점수"), index=1 ("인덱스")) -> (w703:i32[])
                  }
                  frame 1 {
                    n194 = Replace Array Subset(array=w708, new element=2412 ("현점수"), index=1 ("인덱스")) -> (w707:i32[])
                  }
                  frame 2 {
                    n195 = Replace Array Subset(array=w712, new element=3447 ("현점수"), index=1 ("인덱스")) -> (w711:i32[])
                  }
                  frame 3 {
                    n196 = Replace Array Subset(array=w716, new element=3454 ("현점수"), index=1 ("인덱스")) -> (w715:i32[])
                  }
                }
              }
              frame 1 {
                n197 = Replace Array Subset(array=w722, new element=2508 ("현점수"), index=0 ("인덱스")) -> (w719:i32[])
                n198 = case shown="1" w720 {
                  tunnel: w719 -> [w726 w730 w734 w738]
                  tunnel: [w725 w729 w733 w737] -> w718
                  frame 0, Default {
                    n199 = Replace Array Subset(array=w726, new element=3951 ("현점수"), index=1 ("인덱스")) -> (w725:i32[])
                  }
                  frame 1 {
                    n200 = Replace Array Subset(array=w730, new element=2412 ("현점수"), index=1 ("인덱스")) -> (w729:i32[])
                  }
                  frame 2 {
                    n201 = Replace Array Subset(array=w734, new element=3447 ("현점수"), index=1 ("인덱스")) -> (w733:i32[])
                  }
                  frame 3 {
                    n202 = Replace Array Subset(array=w738, new element=3454 ("현점수"), index=1 ("인덱스")) -> (w737:i32[])
                  }
                }
              }
              frame 2 {
                n203 = Replace Array Subset(array=w743, new element=3543 ("현점수"), index=0 ("인덱스")) -> (w742:i32[])
                n204 = case shown="1" w740 {
                  tunnel: w742 -> [w748 w752 w756 w760]
                  tunnel: [w747 w751 w755 w759] -> w741
                  frame 0, Default {
                    n205 = Replace Array Subset(array=w748, new element=3951 ("현점수"), index=1 ("인덱스")) -> (w747:i32[])
                  }
                  frame 1 {
                    n206 = Replace Array Subset(array=w752, new element=2412 ("현점수"), index=1 ("인덱스")) -> (w751:i32[])
                  }
                  frame 2 {
                    n207 = Replace Array Subset(array=w756, new element=3447 ("현점수"), index=1 ("인덱스")) -> (w755:i32[])
                  }
                  frame 3 {
                    n208 = Replace Array Subset(array=w760, new element=3454 ("현점수"), index=1 ("인덱스")) -> (w759:i32[])
                  }
                }
              }
              frame 3 {
                n209 = Replace Array Subset(array=w765, new element=3550 ("현점수"), index=0 ("인덱스")) -> (w764:i32[])
                n210 = case shown="1" w762 {
                  tunnel: w764 -> [w770 w774 w778 w782]
                  tunnel: [w769 w773 w777 w781] -> w763
                  frame 0, Default {
                    n211 = Replace Array Subset(array=w770, new element=3951 ("현점수"), index=1 ("인덱스")) -> (w769:i32[])
                  }
                  frame 1 {
                    n212 = Replace Array Subset(array=w774, new element=2412 ("현점수"), index=1 ("인덱스")) -> (w773:i32[])
                  }
                  frame 2 {
                    n213 = Replace Array Subset(array=w778, new element=3447 ("현점수"), index=1 ("인덱스")) -> (w777:i32[])
                  }
                  frame 3 {
                    n214 = Replace Array Subset(array=w782, new element=3454 ("현점수"), index=1 ("인덱스")) -> (w781:i32[])
                  }
                }
              }
              frame 4 {
                n215 = Replace Array Subset(array=w787, new element=3036 ("현점수"), index=0 ("인덱스")) -> (w786:i32[])
                n216 = case shown="1" w784 {
                  tunnel: w786 -> [w792 w796 w800 w804]
                  tunnel: [w791 w795 w799 w803] -> w785
                  frame 0, Default {
                    n217 = Replace Array Subset(array=w792, new element=3951 ("현점수"), index=1 ("인덱스")) -> (w791:i32[])
                  }
                  frame 1 {
                    n218 = Replace Array Subset(array=w796, new element=2412 ("현점수"), index=1 ("인덱스")) -> (w795:i32[])
                  }
                  frame 2 {
                    n219 = Replace Array Subset(array=w800, new element=3447 ("현점수"), index=1 ("인덱스")) -> (w799:i32[])
                  }
                  frame 3 {
                    n220 = Replace Array Subset(array=w804, new element=3454 ("현점수"), index=1 ("인덱스")) -> (w803:i32[])
                  }
                }
              }
              frame 5 {
                n221 = Replace Array Subset(array=w809, new element=3998 ("현점수"), index=0 ("인덱스")) -> (w808:i32[])
                n222 = case shown="1" w806 {
                  tunnel: w808 -> [w814 w818 w822 w826]
                  tunnel: [w813 w817 w821 w825] -> w807
                  frame 0, Default {
                    n223 = Replace Array Subset(array=w814, new element=3951 ("현점수"), index=1 ("인덱스")) -> (w813:i32[])
                  }
                  frame 1 {
                    n224 = Replace Array Subset(array=w818, new element=2412 ("현점수"), index=1 ("인덱스")) -> (w817:i32[])
                  }
                  frame 2 {
                    n225 = Replace Array Subset(array=w822, new element=3447 ("현점수"), index=1 ("인덱스")) -> (w821:i32[])
                  }
                  frame 3 {
                    n226 = Replace Array Subset(array=w826, new element=3454 ("현점수"), index=1 ("인덱스")) -> (w825:i32[])
                  }
                }
              }
              frame 6 {
                n227 = Replace Array Subset(array=w831, new element=3999 ("현점수"), index=0 ("인덱스")) -> (w830:i32[])
                n228 = case shown="1" w828 {
                  tunnel: w830 -> [w836 w840 w844 w848]
                  tunnel: [w835 w839 w843 w847] -> w829
                  frame 0, Default {
                    n229 = Replace Array Subset(array=w836, new element=3951 ("현점수"), index=1 ("인덱스")) -> (w835:i32[])
                  }
                  frame 1 {
                    n230 = Replace Array Subset(array=w840, new element=2412 ("현점수"), index=1 ("인덱스")) -> (w839:i32[])
                  }
                  frame 2 {
                    n231 = Replace Array Subset(array=w844, new element=3447 ("현점수"), index=1 ("인덱스")) -> (w843:i32[])
                  }
                  frame 3 {
                    n232 = Replace Array Subset(array=w848, new element=3454 ("현점수"), index=1 ("인덱스")) -> (w847:i32[])
                  }
                }
              }
              frame 7 {
                n233 = Replace Array Subset(array=w853, new element=4044 ("현점수"), index=0 ("인덱스")) -> (w852:i32[])
                n234 = case shown="1" w850 {
                  tunnel: w852 -> [w858 w862 w866 w870]
                  tunnel: [w857 w861 w865 w869] -> w851
                  frame 0, Default {
                    n235 = Replace Array Subset(array=w858, new element=3951 ("현점수"), index=1 ("인덱스")) -> (w857:i32[])
                  }
                  frame 1 {
                    n236 = Replace Array Subset(array=w862, new element=2412 ("현점수"), index=1 ("인덱스")) -> (w861:i32[])
                  }
                  frame 2 {
                    n237 = Replace Array Subset(array=w866, new element=3447 ("현점수"), index=1 ("인덱스")) -> (w865:i32[])
                  }
                  frame 3 {
                    n238 = Replace Array Subset(array=w870, new element=3454 ("현점수"), index=1 ("인덱스")) -> (w869:i32[])
                  }
                }
              }
              frame 8 {
                n239 = Replace Array Subset(array=w875, new element=4063 ("현점수"), index=0 ("인덱스")) -> (w874:i32[])
                n240 = case shown="1" w872 {
                  tunnel: w874 -> [w880 w884 w888 w892]
                  tunnel: [w879 w883 w887 w891] -> w873
                  frame 0, Default {
                    n241 = Replace Array Subset(array=w880, new element=3951 ("현점수"), index=1 ("인덱스")) -> (w879:i32[])
                  }
                  frame 1 {
                    n242 = Replace Array Subset(array=w884, new element=2412 ("현점수"), index=1 ("인덱스")) -> (w883:i32[])
                  }
                  frame 2 {
                    n243 = Replace Array Subset(array=w888, new element=3447 ("현점수"), index=1 ("인덱스")) -> (w887:i32[])
                  }
                  frame 3 {
                    n244 = Replace Array Subset(array=w892, new element=3454 ("현점수"), index=1 ("인덱스")) -> (w891:i32[])
                  }
                }
              }
              frame 9 {
                n245 = Replace Array Subset(array=w897, new element=4062 ("현점수"), index=0 ("인덱스")) -> (w896:i32[])
                n246 = case shown="2" w894 {
                  tunnel: w896 -> [w902 w906 w910 w914]
                  tunnel: [w901 w905 w909 w913] -> w895
                  frame 0, Default {
                    n247 = Replace Array Subset(array=w902, new element=3951 ("현점수"), index=1 ("인덱스")) -> (w901:i32[])
                  }
                  frame 1 {
                    n248 = Replace Array Subset(array=w906, new element=2412 ("현점수"), index=1 ("인덱스")) -> (w905:i32[])
                  }
                  frame 2 {
                    n249 = Replace Array Subset(array=w910, new element=3447 ("현점수"), index=1 ("인덱스")) -> (w909:i32[])
                  }
                  frame 3 {
                    n250 = Replace Array Subset(array=w914, new element=3454 ("현점수"), index=1 ("인덱스")) -> (w913:i32[])
                  }
                }
              }
            }
            n251 = And(x=w683, y=w682) -> (x .and. y?=w679:bool)
            n252 = Quotient & Remainder(x=w689, y=2) -> (x-y*floor(x/y)=w687:i32)  [unwired: 1 out]
            n253 = Equal To 0?(x=w687) -> (x = 0?=w686:bool)
            n254 = case shown="참" w679 {
              tunnel: w678 -> [_ w924]
              tunnel: w674 -> [w918 w925]
              tunnel: [w916 w926] -> w680
              frame False {
                n255 = Equal?(x=w918, y=11) -> (x = y?=w917:bool)
                n256 = case shown="참" w917 {
                  tunnel: [컨트롤_2."대기" 컨트롤_2."0세트승리"] -> w916
                  frame False {
                  }
                  frame True {
                  }
                }
              }
              frame True {
                n257 = Subtract(x=w925, y=w924) -> (x-y=w928:i32)
                n258 = Absolute Value(x=w928) -> (abs(x)=w927:i32)
                n259 = Greater Than 0?(x=w928) -> (x > 0?=w931:bool)
                n260 = Greater Or Equal?(x=w927, y=2) -> (x >= y?=w923:bool)
                n261 = And(x=w931, y=w923) -> (x .and. y?=w930:bool)
                n262 = Select(t=컨트롤_2."0세트승리", s=w930, f=컨트롤_2."대기") -> (s? t:f=w926:T1)
              }
            }
            n263 = case shown="거짓" w686 {
              tunnel: w694 -> [w940 w960]
              tunnel: w693 -> [w939 w959]
              tunnel: [w936 w960] -> w685
              tunnel: [w933 w959] -> w692
              tunnel: [w934 w958] -> w671
              tunnel: [w938 w957] -> w668
              tunnel: w670 -> [w937 w957]
              tunnel: w669 -> [w935 w958]
              frame False {
                n264 = Not(x=w940) -> (.not. x?=w936:bool)
                n265 = Not(x=w939) -> (.not. x?=w933:bool)
                n266 = case shown="참" w933 {
                  tunnel: [w946 w954] -> w938
                  tunnel: w937 -> [w945 w953]
                  tunnel: w935 -> [w942 w950]
                  tunnel: [w941 w949] -> w934
                  frame False {
                    n267 = Replace Array Subset(array=w942, new element=u32 4096 ("Waveform"), index=0 ("인덱스")) -> (w941:u32[])
                    n268 = Replace Array Subset(array=w945, new element=u32 0 ("새 원소/부분배열"), index=0 ("인덱스")) -> (w946:u32[])
                  }
                  frame True {
                    n269 = Replace Array Subset(array=w953, new element=u32 32768 ("새 원소/부분배열"), index=0 ("인덱스")) -> (w954:u32[])
                    n270 = Replace Array Subset(array=w950, new element=u32 0 ("Waveform"), index=0 ("인덱스")) -> (w949:u32[])
                  }
                }
              }
              frame True {
              }
            }
          }
          frame True {
            w969 = FALSE
          }
        }
      }
      frame "0세트승리" {
        w987 = FALSE
        n271 = local read "Elapsed Time (s) 5"() -> (w978:dbl)
        n272 = Greater?(x=w978, y=2) -> (0:w984:bool)
        n273 = call "경과 시간6"("Reset"=w984) -> ("Elapsed Time (s)"=→"Elapsed Time (s) 5":dbl, "Time has Elapsed"=w983:bool)  [unwired: 11 in, 6 out]
        n274 = case shown="참" w983 {
          tunnel: w994 -> [w998 w1005]
          tunnel: [w998 w1004] -> w992
          tunnel: [컨트롤_2."0세트승리" w1007] -> w991
          tunnel: [w999 w1006] -> w986
          tunnel: w981 -> [w999 _]
          tunnel: w980 -> [w995 _]
          tunnel: [w995 w1006] -> w979
          tunnel: w977 -> [w997 w1003]
          tunnel: [w997 w1002] -> w976
          tunnel: [w996 w1001] -> w972
          tunnel: w971 -> [w996 _]
          frame False {
          }
          frame True {
            w1001 = i32[] [4047, 3951, 3823, 2031]  # 점수
            w1006 = 0
            n275 = Increment(x=w1005) -> (x+1=w1004:i32)
            n276 = case shown="2" w1004 {
              tunnel: w1003 -> [w1012 w1016 w1018]
              tunnel: [w1012 w1013 w1017] -> w1002
              frame 0, Default {
              }
              frame 1 {
                n277 = Replace Array Subset(array=w1016, new element=u32 30976 ("새 원소/부분배열"), index=0 ("인덱스")) -> (w1013:u32[])
              }
              frame 2 {
                n278 = Replace Array Subset(array=w1018, new element=u32 9216 ("새 원소/부분배열"), index=0 ("인덱스")) -> (w1017:u32[])
              }
            }
            n279 = Equal?(x=w1004, y=2) -> (x = y?=w1011:bool)
            n280 = Select(t=컨트롤_2."경기끝!", s=w1011, f=컨트롤_2."대기") -> (s? t:f=w1007:T1)
          }
        }
      }
      frame "1세트승리" {
        w1028 = FALSE
        n281 = local read "Elapsed Time (s) 3"() -> (w1029:dbl)
        n282 = Greater?(x=w1029, y=2) -> (0:w1032:bool)
        n283 = call "경과 시간5"("Reset"=w1032) -> ("Elapsed Time (s)"=→"Elapsed Time (s) 3":dbl, "Time has Elapsed"=w1031:bool)  [unwired: 11 in, 6 out]
        n284 = case shown="거짓" w1031 {
          tunnel: w1043 -> [w1048 w1061]
          tunnel: [w1048 w1054] -> w1042
          tunnel: [컨트롤_2."1세트승리" w1060] -> w1041
          tunnel: [w1050 w1059] -> w1037
          tunnel: [w1049 w1059] -> w1036
          tunnel: w1035 -> [w1050 _]
          tunnel: w1034 -> [w1049 _]
          tunnel: w1027 -> [w1046 w1053]
          tunnel: [w1046 w1052] -> w1026
          tunnel: [w1045 w1051] -> w1022
          tunnel: w1021 -> [w1045 _]
          frame False {
          }
          frame True {
            w1051 = i32[] [4047, 3951, 3823, 2031]  # 점수
            w1059 = 0
            n285 = Increment(x=w1061) -> (x+1=w1054:i32)
            n286 = case shown="2" w1054 {
              tunnel: w1053 -> [w1062 w1064 w1068]
              tunnel: [w1062 w1063 w1067] -> w1052
              frame 0, Default {
              }
              frame 1 {
                n287 = Replace Array Subset(array=w1064, new element=u32 243 ("새 원소/부분배열"), index=0 ("인덱스")) -> (w1063:u32[])
              }
              frame 2 {
                n288 = Replace Array Subset(array=w1068, new element=u32 73 ("새 원소/부분배열"), index=0 ("인덱스")) -> (w1067:u32[])
              }
            }
            n289 = Equal?(x=w1054, y=2) -> (x = y?=w1058:bool)
            n290 = Select(t=컨트롤_2."경기끝!", s=w1058, f=컨트롤_2."대기") -> (s? t:f=w1060:T1)
          }
        }
      }
      frame "경기끝!" {
        n291 = Equal?(x=w1078, y=2) -> (x = y?=w1076:bool)
        n292 = case shown="거짓" w1076 {
          tunnel: [FALSE TRUE] -> w1080
          tunnel: [TRUE FALSE] -> w1079
          frame False {
          }
          frame True {
          }
        }
        n293 = call "사용자에게 메시지 디스플레이"() -> ()  [unwired: 10 in, 2 out]
      }
    }
    "1현점수" <- w39
    "0현점수" <- w40
    "player 2" <- w37
    "player 1" <- w38
    "몇번째 경기" <- w105
    "0세트점수" <- w34
    "1세트점수" <- w41
    n294 = Unbundle By Name(w136) -> ("status"=w135:bool)
    n295 = Or(x=w135, y="RESET") -> (x .or. y?=w36:bool)
    n296 = Select(t=w102, s=w101, f=w94) -> (s? t:f=w103:i32)
    "0터치횟수" <- w103
    n297 = Select(t=w102, s=w101, f=w95) -> (s? t:f=w100:i32)
    "1터치횟수" <- w100
    n298 = Or(x=w36, y=w97) -> (x .or. y?=w96:bool)
    n299 = Bundle By Name(cluster=w108, "LED1차례"=w67, "1세트 이진수점수"=w73, "0세트 이진수점수"=w76, "점수"=w82, "몇번째 경기"=w105, "LED0"=w37, "LED1"=w38, "0번터치 횟수"=w103, "1번터치 횟수"=w100, "0현점수"=w40, "1현점수"=w39, "0세트점수"=w34, "1세트점수"=w41, "LED0차례"=w64) -> (w118:T2)
    n300 = Index Array(array=w67, index=0 ("인덱스")) -> (element=w65:u32)
    n301 = Index Array(array=w73, index=0 ("인덱스")) -> (element=w77:u32)
    n302 = Index Array(array=w76, index=0 ("인덱스")) -> (element=w74:u32)
    n303 = Not Equal?(x=w85, y=컨트롤_2."대기") -> (x != y?=w83:bool)
    n304 = Compound Arithmetic op=ADD(w65, w74, w77) -> (w71:u32)
    n305 = call <vilib>:"DAQmx Is Task Done.vi"("task/channels in"=w126, "error in"=w81) -> ("task out"=w132:refnum<k21>, "error out"=w131:errorcluster)  [unwired: 11 in, 1 out]
    n306 = call "경과 시간9"("Reset"=w83) -> ("Elapsed Time (s)"=→"Elapsed Time (s) 9":dbl, "Time has Elapsed"=w87:bool)  [unwired: 11 in, 6 out]
    n307 = Replace Array Subset(array=u32[] [16513] ("배열"), new element=w71, index=0 ("인덱스")) -> (w69:u32[])
    n308 = shared-variable "내 컴퓨터\\ipad.lvlib\\set1"(w34) -> ()  [unwired: 1 in, 1 out]
    n309 = shared-variable "내 컴퓨터\\ipad.lvlib\\score0"(w40) -> ()  [unwired: 1 in, 1 out]
    n310 = shared-variable "내 컴퓨터\\ipad.lvlib\\serve0"(w37) -> ()  [unwired: 1 in, 1 out]
    n311 = shared-variable "내 컴퓨터\\ipad.lvlib\\serve1"(w38) -> ()  [unwired: 1 in, 1 out]
    n312 = shared-variable "내 컴퓨터\\ipad.lvlib\\set0"(w34) -> ()  [unwired: 1 in, 1 out]
    n313 = call "DAQ 어시스턴트"("data"=w69) -> ()  [unwired: 17 in, 2 out]
    n314 = Select(t=컨트롤_2."경기끝!", s=w87, f=w85) -> (s? t:f=w88:T1)
    n315 = shared-variable "내 컴퓨터\\ipad.lvlib\\score1"(w39) -> ()  [unwired: 1 in, 1 out]
  }
  n316 = call <vilib>:"DAQmx Stop Task.vi"("task/channels in"=w18, "error in"=w16) -> ("task out"=w17:refnum<k21>, "error out"=w20:errorcluster)  [unwired: 12 in]
  n317 = call <vilib>:"DAQmx Clear Task.vi"("task in"=w8, "error in"=w7) -> ("error out"=w9:errorcluster)  [unwired: 13 in]
  n318 = case shown="참" w2 {
    frame False {
    }
    frame True {
      n319 = control-ref of="이 VI"() -> (w1098:refnum<vi>)
      n320 = invoke class="VI" method="Default Vals.Reinit All"(reference=w1098) -> ()  [unwired: 2 in, 3 out]
    }
  }
  n321 = call <vilib>:"Simple Error Handler.vi"("error in (no error)"=w9) -> ()  [unwired: 4 in, 5 out]
  n322 = call <vilib>:"DAQmx Clear Task.vi"("task in"=w17, "error in"=w20) -> ("error out"=w19:errorcluster)  [unwired: 13 in]
  n323 = call <vilib>:"Simple Error Handler.vi"("error in (no error)"=w19) -> ()  [unwired: 4 in, 5 out]
